vi "Go.vi"(9 "Timing Data":T1(array[cluster]), 10 "Control In":T2={"I-O.lvclass"=refnum, "Gantry"=refnum, "Dispenser"="COM1"}, 11 "Sensor Dispense in":refnum<class "Sensor Dispense.lvclass">) -> (2 "Control Out":T2={"I-O.lvclass"=refnum, "Gantry"=refnum, "Dispenser"="COM1"}, 3 "Sensor Dispense out":refnum<class "Sensor Dispense.lvclass">)   [LabVIEW 2021, in "Sensor Dispense.lvclass"]
uses:
  Sensor Dispense.lvclass
  C:/Users/HEP/Documents/GitHub/Gantry/UCSB-Gantry-HEP-main/Classes/Routine/Dispense/Dispense.lvclass
  Classes/Controller/Controllers.ctl
  Classes/Controller/I-O/I-O.lvclass
  C:/Program Files (x86)/Aerotech/A3200/LabVIEW/2010/Bin/Aerotech.A3200.dll
  Program Files (x86)/Aerotech/A3200/LabVIEW/2010/Bin/Aerotech.A3200.dll
  Sensor Dispense.lvclass/Sensor Dispense.ctl
  Classes/Controller/Motion/Motion.lvclass
  Classes/Controller/Dispenser/Dispenser.lvclass
  Classes/Controller/Motion/A3200/A3200.lvclass
  Classes/Controller/Controller.lvclass
panel:
  out "error out":errorcluster
  in  "error in (no error)":errorcluster
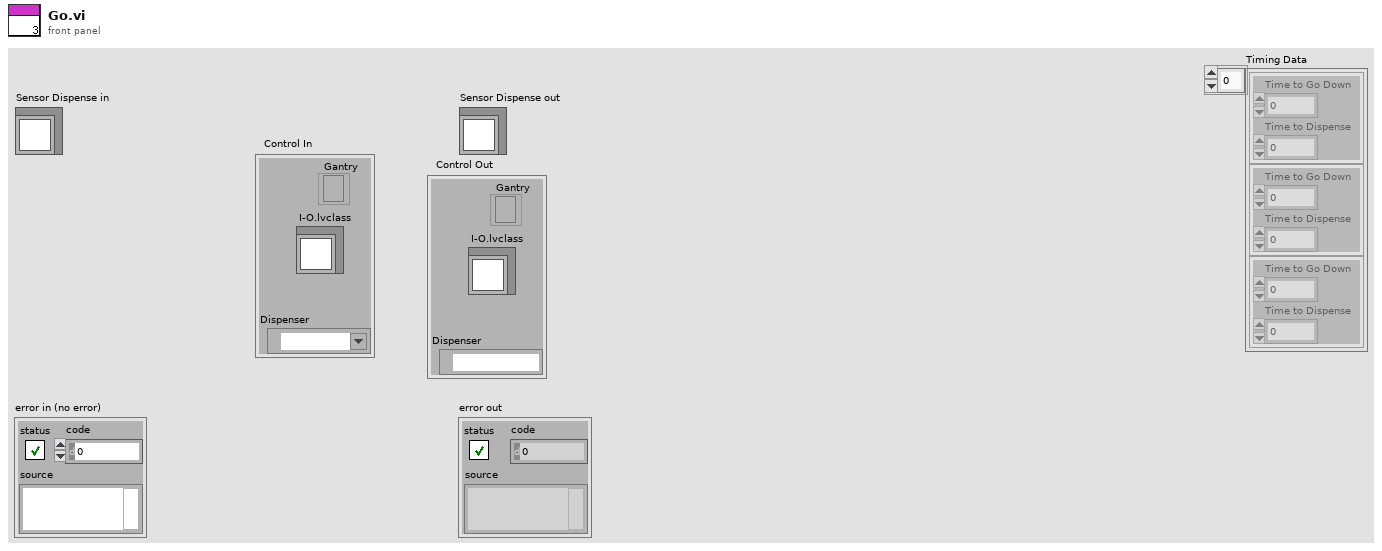
[diagram p1: front panel]
types:
  T1 = cluster{"Time to Go Down":i32, "Time to Dispense":i32}[]
  T2 = typedef "Controller.lvclass/Controllers.ctl" = cluster{"I-O.lvclass":refnum<class "I-O.lvclass">, "Gantry":refnum<k24>, "Dispenser":refnum<visa-resource-name>}
  T3 = cluster{"Endpoints":dbl[][], "Center":dbl[], "CW/CCW":dbl, "Dispense Type":enum16{"N-gon", "Square", "Arc", "Dot", "Line", "Circle"}}[]
  T4 = cluster{"Endpoints":dbl[][], "Center":dbl[], "CW/CCW":dbl, "Dispense Type":enum16{"N-gon", "Square", "Arc", "Dot", "Line", "Circle"}}
  T5 = enum16{"N-gon", "Square", "Arc", "Dot", "Line", "Circle"}
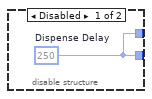
[diagram p2: hidden frame]
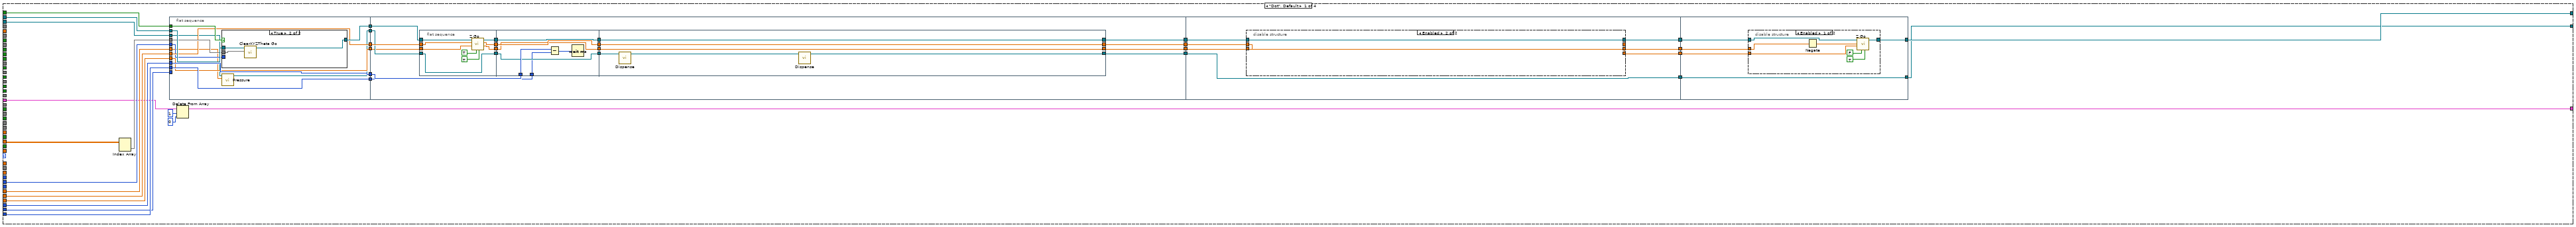
[diagram p4: hidden frame]
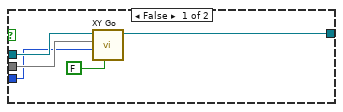
[diagram p5: hidden frame]
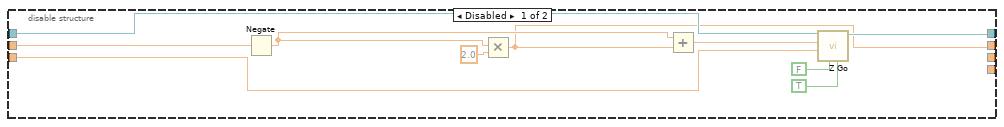
[diagram p6: hidden frame]
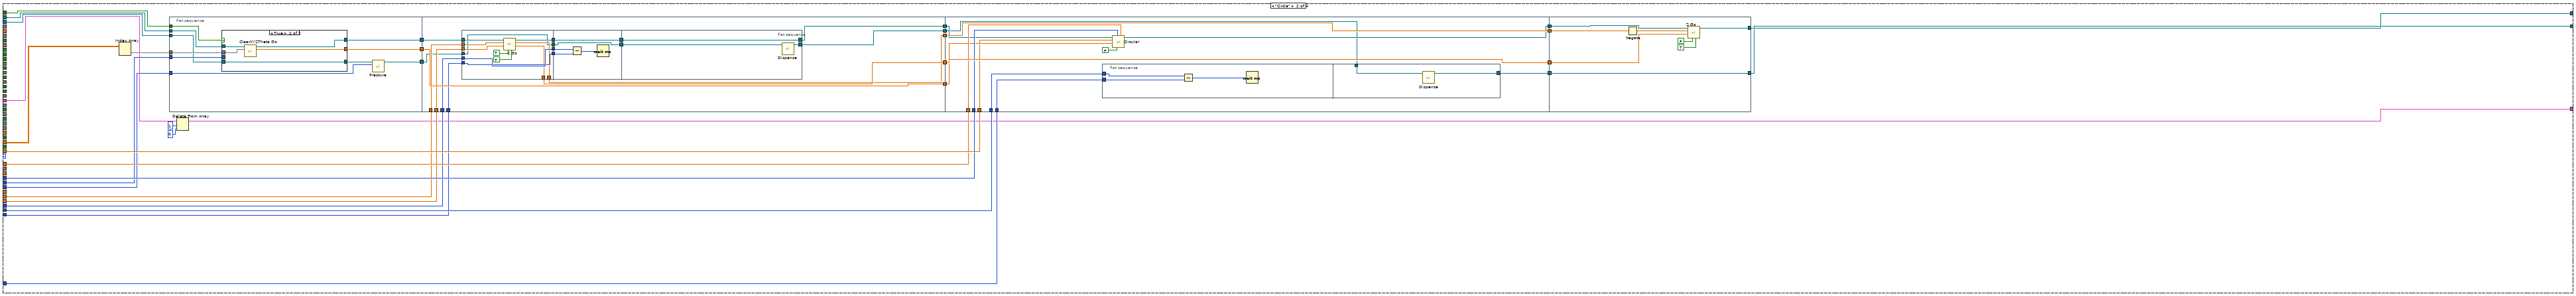
[diagram p8: hidden frame]
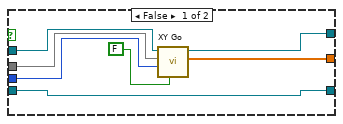
[diagram p9: hidden frame]
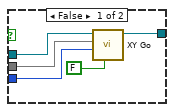
[diagram p10: hidden frame]
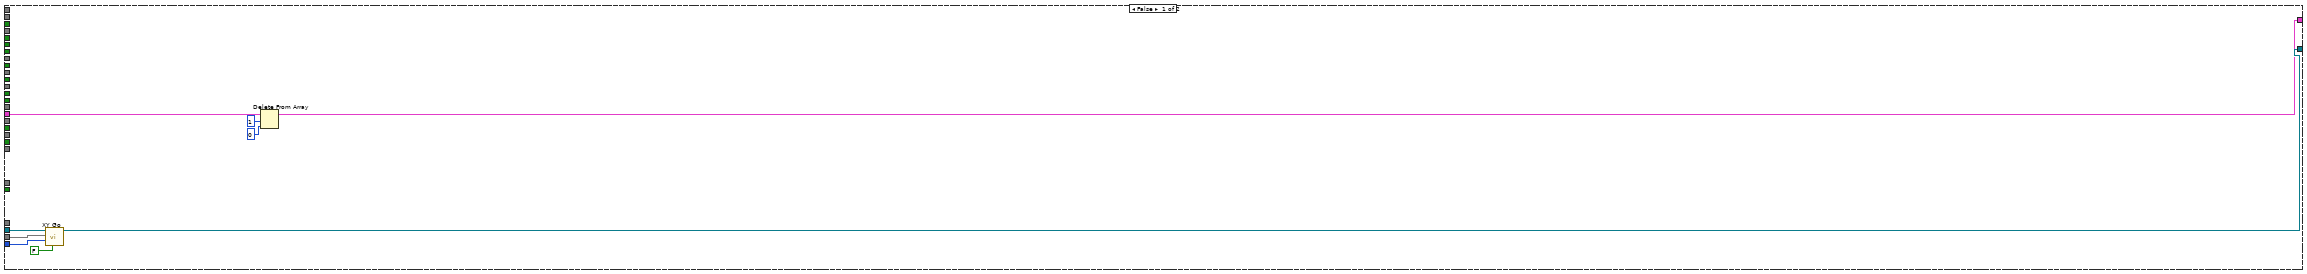
[diagram p11: hidden frame]
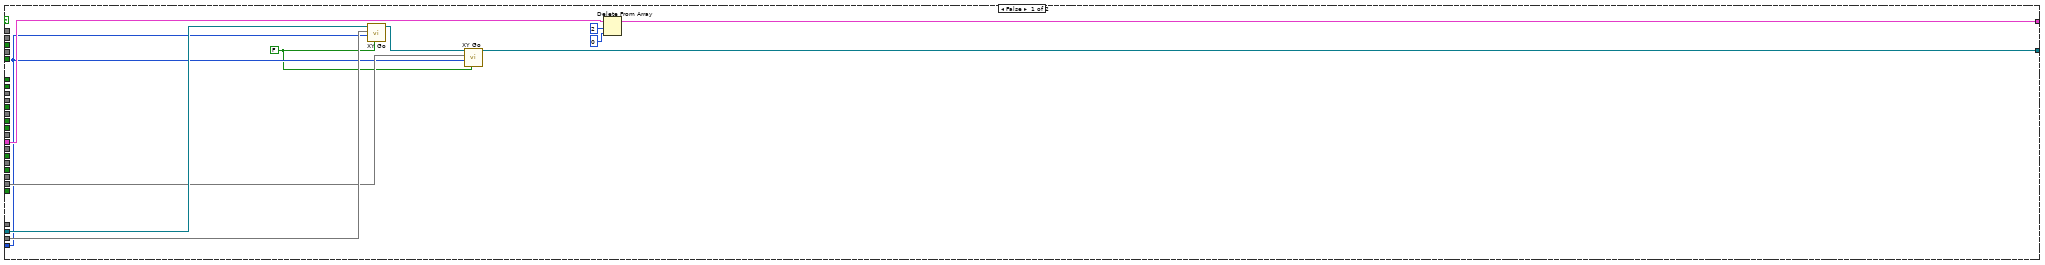
[diagram p12: hidden frame]
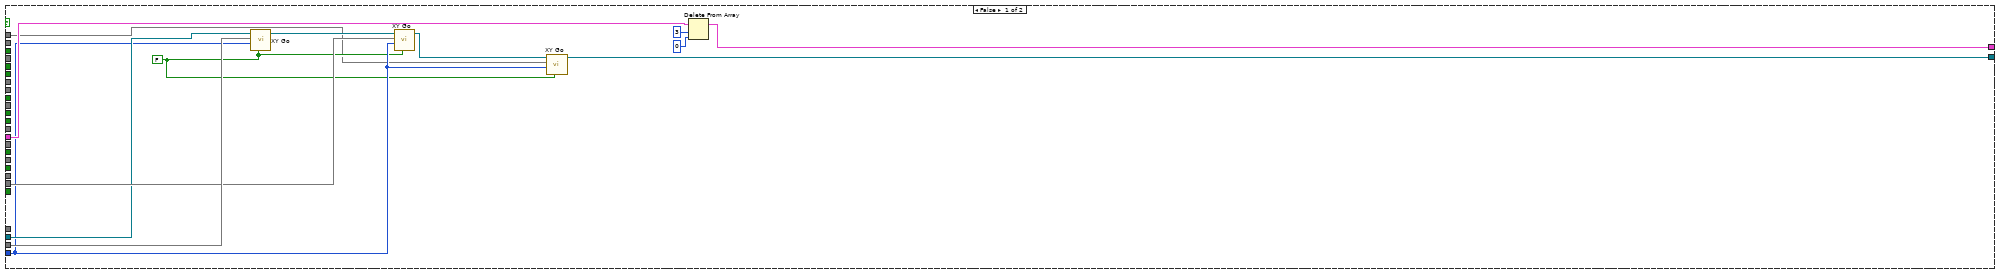
[diagram p13: hidden frame]
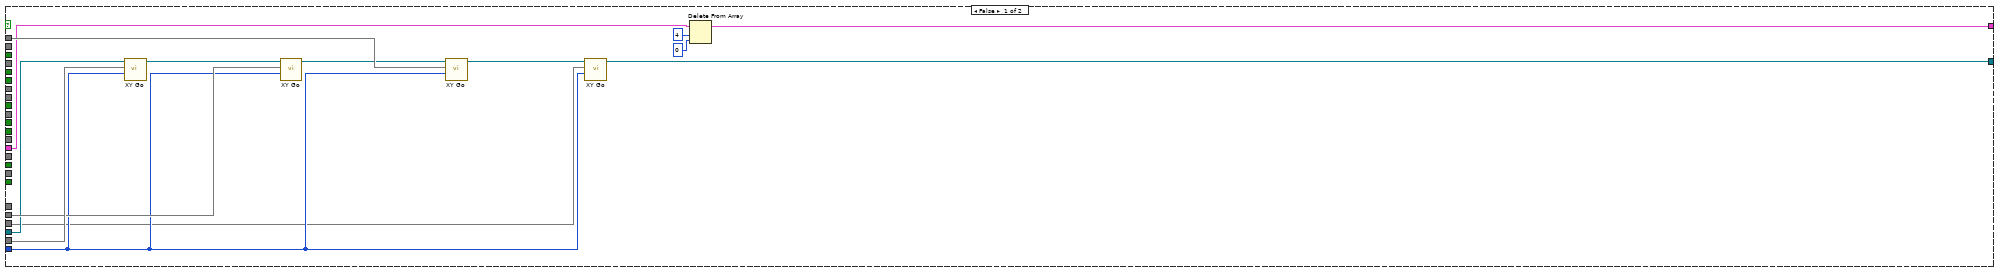
[diagram p14: hidden frame]
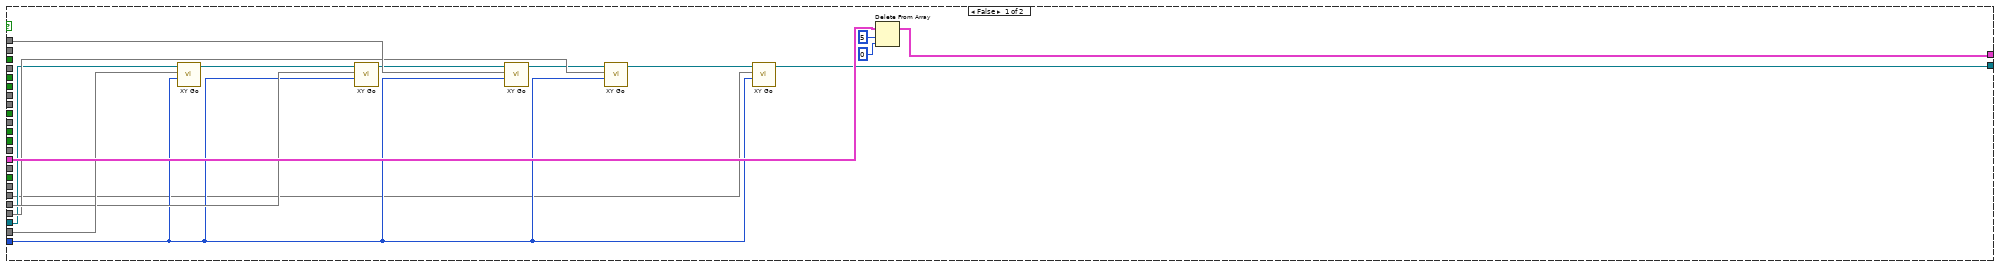
[diagram p15: hidden frame]
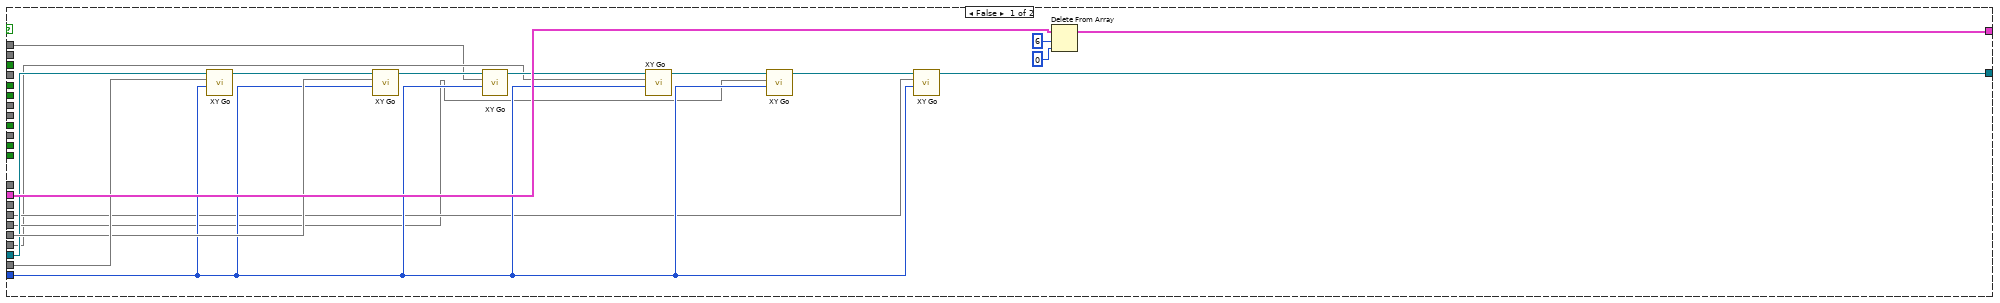
[diagram p16: hidden frame]
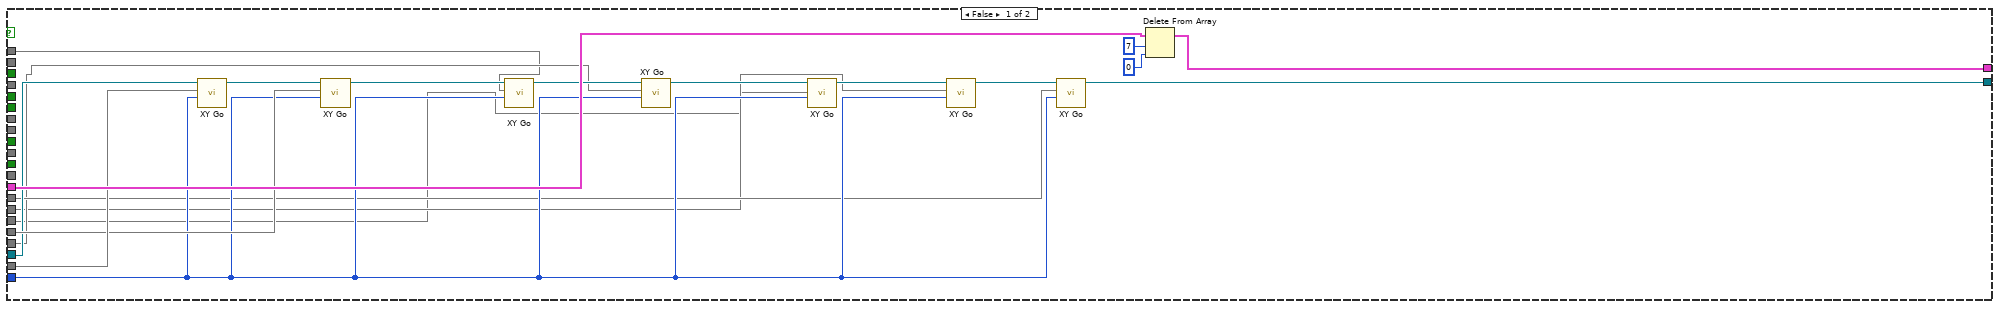
[diagram p17: hidden frame]
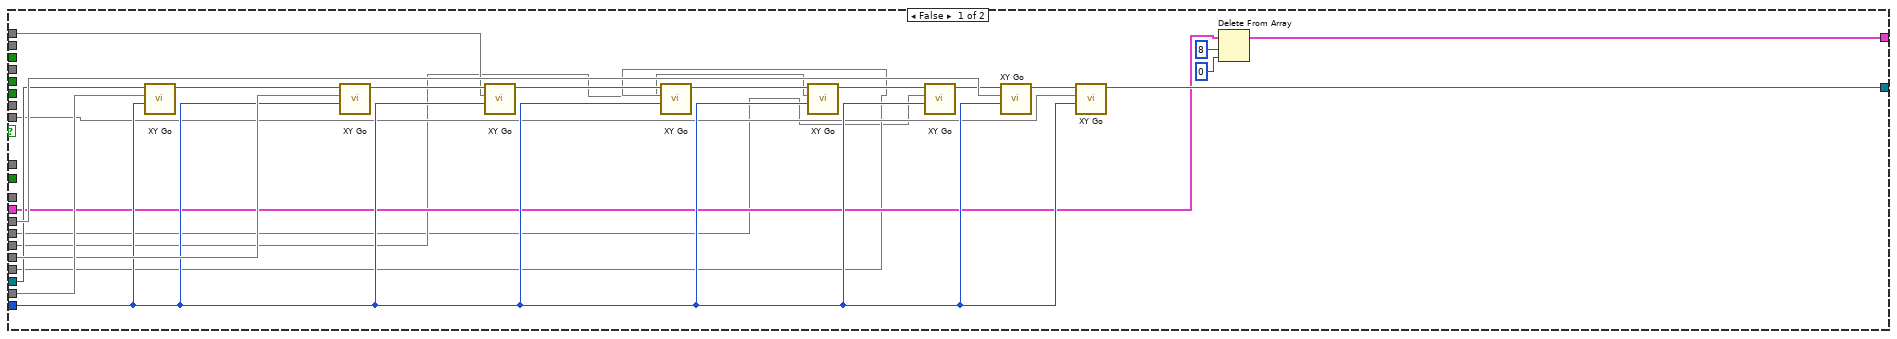
[diagram p18: hidden frame]
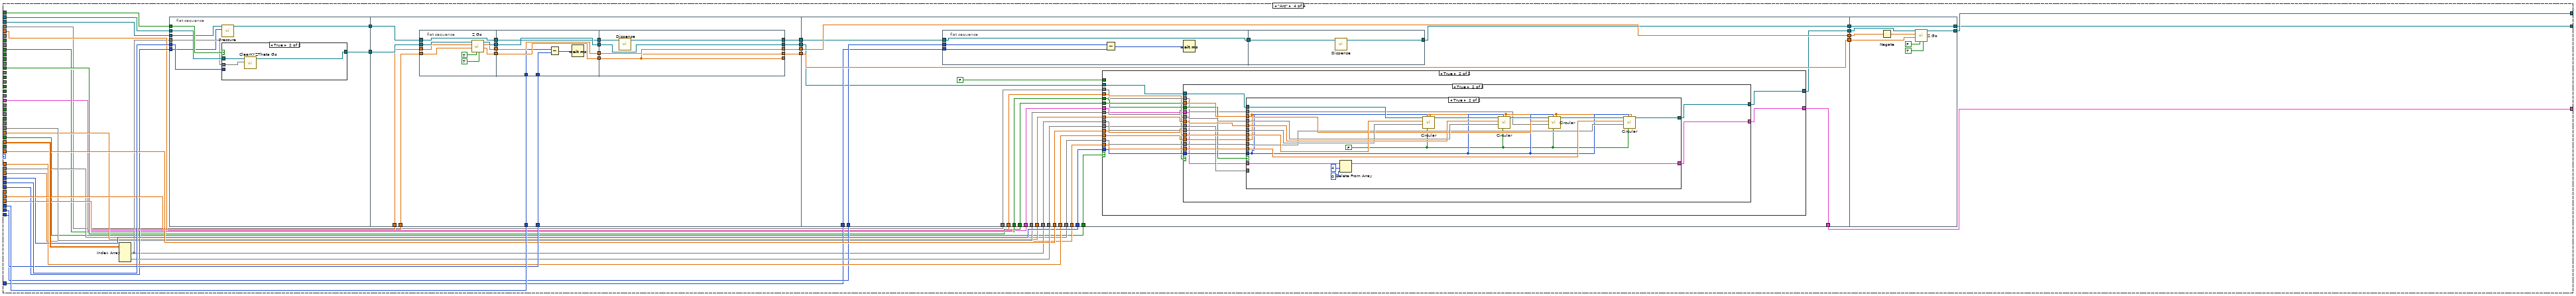
[diagram p19: hidden frame]
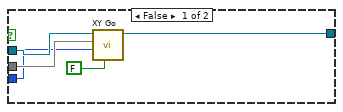
[diagram p20: hidden frame]
diagram:
  n1 = case shown="No Error" "error in (no error)" {
    selector: "error in (no error)" -> [w7 w1391]
    tunnel: "Sensor Dispense in" -> [w12 w1390]
    tunnel: [w11 w1390] -> w5
    tunnel: "Control In" -> [w10 w1389]
    tunnel: [w9 w1389] -> w3
    tunnel: [w8 w1391] -> w2
    frame No Error {
      n2 = in-place {
        in-place-border: w12 -> [w24]
        in-place-border: [w23] -> w11
        in-place-border: w7 -> [w17]
        in-place-border: [w16] -> w8
        n3 = in-place-cluster #1(w10) -> ("Gantry"=w25:refnum<k24>, "Dispenser"=w20:refnum<visa-resource-name>)
        n4 = Unbundle By Name(w24) -> ("Dispense Steps"=w21:T3, "Glue Speed"=w15:i32, "Move Speed"=w26:i32, "Line Pressure"=w13:i64, "Dot Pressure"=w14:dbl)
        n5 = while {
          tunnel: w26 -> [w167]
          shift-right: [w159] -> w22
          shift-left: w25 -> [w165]
          tunnel: w15 -> [w166]
          shift-right: [w151] -> w23
          shift-left: w24 -> [w163]
          shift-right: [w154] -> w18
          shift-left: w20 -> [w157]
          tunnel: "Timing Data" -> [w156] mode=indexing
          shift-right: [w147] -> w16
          shift-left: w17 -> [w147]
          tunnel: w14 -> [w149]
          tunnel: w13 -> [w148]
          shift-right: [w111] -> _
          shift-left: w21 -> [w63]
          i -> [w162]
          stop <- w113 stop-if-true
          # "740 is good"
          # "compares 3 and 4"
          # "compares 2 and 3"
          # "Compares 1 and 2"
          # "#2"
          # "#3"
          # "#4"
          # "#3"
          # "1/11/23 - Originally 750"
          n6 = Unbundle By Name(w156) -> ("Time to Go Down"=w155:i32, "Time to Dispense"=w145:i32)
          n7 = disable-structure shown="Enabled" {
            disable-tunnel: [w168 w172] -> w150
            disable-tunnel: [w168 w170] -> w146
            disable-tunnel: w145 -> [_ w171]
            frame Disabled {
              w168 = 250  # Dispense Delay
            }
            frame Enabled {
              w169 = 450  # End Dispense Delay
              w172 = 740  # Start Dispense Delay
              # "For arcs it is set to 250"
              # "525 - 1/23/2023"
              # "Originally 0"
              n8 = disable-structure shown="Disabled" {
                disable-tunnel: w171 -> [w177 _]
                disable-tunnel: [w174 w178] -> w170
                disable-tunnel: w169 -> [w173 w178]
                frame Disabled {
                  n9 = Less?(x=w177, y=w173) -> (x < y?=w176:bool)
                  n10 = Select(t=0, s=w176, f=w173) -> (s? t:f=w174:i32)
                }
                frame Enabled {
                }
              }
            }
          }
          n11 = Index Array(array=w63) -> (element=w143:T4)  [unwired: 1 in]
          n12 = Index Array(array=w63, index=11) -> (element=w69:T4)
          n13 = Index Array(array=w63, index=7) -> (element=w104:T4)
          n14 = Index Array(array=w63, index=9) -> (element=w75:T4)
          n15 = Index Array(array=w63, index=10) -> (element=w72:T4)
          n16 = Index Array(array=w63, index=12) -> (element=w66:T4)
          n17 = Index Array(array=w63, index=2) -> (element=w140:T4)
          n18 = Index Array(array=w63, index=8) -> (element=w78:T4)
          n19 = Index Array(array=w63, index=4) -> (element=w110:T4)
          n20 = Index Array(array=w63, index=6) -> (element=w106:T4)
          n21 = Index Array(array=w63, index=5) -> (element=w108:T4)
          n22 = Index Array(array=w63, index=1) -> (element=w142:T4)
          n23 = Index Array(array=w63, index=3) -> (element=w139:T4)
          n24 = Unbundle By Name(w140) -> ("Endpoints"=w137:dbl[][], "Center"=w118:dbl[])
          n25 = Unbundle By Name(w75) -> ("Endpoints"=w74:dbl[][])  [unwired: 1 out]
          n26 = Unbundle By Name(w104) -> ("Endpoints"=w103:dbl[][])  [unwired: 1 out]
          n27 = Unbundle By Name(w78) -> ("Endpoints"=w77:dbl[][])  [unwired: 1 out]
          n28 = Unbundle By Name(w110) -> ("Endpoints"=w109:dbl[][])  [unwired: 1 out]
          n29 = Unbundle By Name(w143) -> ("Endpoints"=w134:dbl[][], "Center"=w158:dbl[], "Dispense Type"=w160:T5, "CW/CCW"=w164:dbl)
          n30 = Unbundle By Name(w106) -> ("Endpoints"=w105:dbl[][])  [unwired: 1 out]
          n31 = Unbundle By Name(w139) -> ("Endpoints"=w138:dbl[][], "Center"=w117:dbl[])
          n32 = Unbundle By Name(w108) -> ("Endpoints"=w107:dbl[][])  [unwired: 1 out]
          n33 = Unbundle By Name(w142) -> ("Endpoints"=w141:dbl[][], "Center"=w119:dbl[])
          n34 = Unbundle By Name(w69) -> ("Endpoints"=w68:dbl[][])  [unwired: 1 out]
          n35 = Unbundle By Name(w72) -> ("Endpoints"=w71:dbl[][])  [unwired: 1 out]
          n36 = Unbundle By Name(w66) -> ("Endpoints"=w65:dbl[][])  [unwired: 1 out]
          n37 = Index Array(array=w103) -> (element #1=w82:dbl[], element #2=w61:dbl[])  [unwired: 4 in]
          n38 = Index Array(array=w137) -> (element #1=w131:dbl[], element #2=w27:dbl[])  [unwired: 4 in]
          n39 = Index Array(array=w107) -> (element #1=w93:dbl[], element #2=w31:dbl[])  [unwired: 4 in]
          n40 = Index Array(array=w138) -> (element #1=w130:dbl[], element #2=w28:dbl[])  [unwired: 4 in]
          n41 = Index Array(array=w77) -> (element #1=w62:dbl[], element #2=w55:dbl[])  [unwired: 4 in]
          n42 = Index Array(array=w74) -> (element #1=w56:dbl[], element #2=w49:dbl[])  [unwired: 4 in]
          n43 = Index Array(array=w109) -> (element #1=w98:dbl[], element #2=w30:dbl[])  [unwired: 4 in]
          n44 = Index Array(array=w105) -> (element #1=w88:dbl[], element #2=w29:dbl[])  [unwired: 4 in]
          n45 = Index Array(array=w141) -> (element #1=w132:dbl[], element #2=w120:dbl[])  [unwired: 4 in]
          n46 = Index Array(array=w68) -> (element #1=w43:dbl[], element #2=w38:dbl[])  [unwired: 4 in]
          n47 = Index Array(array=w71) -> (element #1=w50:dbl[], element #2=w44:dbl[])  [unwired: 4 in]
          n48 = Index Array(array=w65) -> (element #1=w37:dbl[], element #2=w32:dbl[])  [unwired: 4 in]
          n49 = Index Array(array=w134) -> (element #2=w133:dbl[])  [unwired: 4 in, 1 out]
          n50 = Equal?(x=w38, y=w37) -> (x = y?=w36:bool[])
          n51 = Equal?(x=w44, y=w43) -> (x = y?=w42:bool[])
          n52 = Equal?(x=w49, y=w50) -> (x = y?=w48:bool[])
          n53 = Equal?(x=w120, y=w131) -> (x = y?=w126:bool[])
          n54 = Equal?(x=w61, y=w62) -> (x = y?=w60:bool[])
          n55 = Equal?(x=w55, y=w56) -> (x = y?=w54:bool[])
          n56 = Equal?(x=w29, y=w82) -> (x = y?=w83:bool[])
          n57 = Equal?(x=w31, y=w88) -> (x = y?=w87:bool[])
          n58 = Equal?(x=w30, y=w93) -> (x = y?=w92:bool[])
          n59 = Equal?(x=w28, y=w98) -> (x = y?=w97:bool[])
          n60 = Equal?(x=w27, y=w130) -> (x = y?=w125:bool[])
          n61 = Index Array(array=w125) -> (element #1=w122:bool, element #2=w121:bool)  [unwired: 2 in]
          n62 = And(x=w122, y=w121) -> (x .and. y?=w114:bool)
          n63 = Index Array(array=w36) -> (element #1=w35:bool, element #2=w34:bool)  [unwired: 2 in]
          n64 = Equal?(x=w133, y=w132) -> (x = y?=w129:bool[])
          n65 = Index Array(array=w48) -> (element #1=w47:bool, element #2=w46:bool)  [unwired: 2 in]
          n66 = Index Array(array=w126) -> (element #1=w124:bool, element #2=w123:bool)  [unwired: 2 in]
          n67 = Index Array(array=w60) -> (element #1=w59:bool, element #2=w58:bool)  [unwired: 2 in]
          n68 = Index Array(array=w54) -> (element #1=w53:bool, element #2=w52:bool)  [unwired: 2 in]
          n69 = Index Array(array=w83) -> (element #1=w81:bool, element #2=w80:bool)  [unwired: 2 in]
          n70 = Index Array(array=w87) -> (element #1=w86:bool, element #2=w85:bool)  [unwired: 2 in]
          n71 = Index Array(array=w92) -> (element #1=w91:bool, element #2=w90:bool)  [unwired: 2 in]
          n72 = property on="Property Node" class="Sensor Dispense.lvclass"(reference=w163) -> (reference out=w151:refnum<class "Sensor Dispense.lvclass">, "Z height"=w153:dbl, "Z speed"=w152:dbl)  [unwired: 1 in, 1 out]
          n73 = Index Array(array=w42) -> (element #1=w41:bool, element #2=w40:bool)  [unwired: 2 in]
          n74 = Index Array(array=w97) -> (element #1=w96:bool, element #2=w95:bool)  [unwired: 2 in]
          n75 = And(x=w35, y=w34) -> (x .and. y?=w33:bool)
          n76 = Index Array(array=w129) -> (element #1=w128:bool, element #2=w127:bool)  [unwired: 2 in]
          n77 = And(x=w41, y=w40) -> (x .and. y?=w39:bool)
          n78 = And(x=w47, y=w46) -> (x .and. y?=w45:bool)
          n79 = And(x=w59, y=w58) -> (x .and. y?=w57:bool)
          n80 = And(x=w53, y=w52) -> (x .and. y?=w51:bool)
          n81 = And(x=w81, y=w80) -> (x .and. y?=w79:bool)
          n82 = And(x=w86, y=w85) -> (x .and. y?=w84:bool)
          n83 = And(x=w91, y=w90) -> (x .and. y?=w89:bool)
          n84 = And(x=w96, y=w95) -> (x .and. y?=w94:bool)
          n85 = And(x=w124, y=w123) -> (x .and. y?=w115:bool)
          n86 = And(x=w128, y=w127) -> (x .and. y?=w116:bool)
          n87 = Equal To 0?(x=w162) -> (x = 0?=w161:bool)
          n88 = case shown="\"Line\"" w160 {
            tunnel: w158 -> [_ w333 _ w1181]
            tunnel: w165 -> [w209 w334 w484 w1189]
            tunnel: w167 -> [w192 w327 w483 w1187]
            tunnel: [w208 w337 w480 w1177] -> w159
            tunnel: w166 -> [_ w332 w471 w1180]
            tunnel: w164 -> [_ w331 _ w1179]
            tunnel: w152 -> [w200 w329 w468 w1183]
            tunnel: w153 -> [w201 w330 w469 w1184]
            tunnel: w161 -> [w210 w328 w482 w1190]
            tunnel: w157 -> [w199 w311 w475 w1173]
            tunnel: w155 -> [w197 w318 w473 w1186]
            tunnel: w145 -> [w202 w319 w470 w1178]
            tunnel: w150 -> [w203 w317 w474 w1185]
            tunnel: [w207 w312 w478 w1176] -> w154
            tunnel: w134 -> [w206 w316 w477 w1188]
            tunnel: w149 -> [w191 _ _ _]
            tunnel: w148 -> [_ w309 w451 w1172]
            tunnel: w146 -> [_ w308 w450 w1171]
            tunnel: w120 -> [_ _ w447 w1170]
            tunnel: w119 -> [_ _ _ w1169]
            tunnel: w118 -> [_ _ _ w1168]
            tunnel: w117 -> [_ _ _ w1166]
            tunnel: w28 -> [_ _ w442 w1165]
            tunnel: w116 -> [_ _ w445 w1164]
            tunnel: w115 -> [_ _ w444 w1163]
            tunnel: w114 -> [_ _ w443 w1162]
            tunnel: w63 -> [w183 w307 w448 w1161]
            tunnel: [w180 w304 w449 w1160] -> w111
            tunnel: w27 -> [_ _ w446 w1159]
            tunnel: w94 -> [_ _ w441 _]
            tunnel: w30 -> [_ _ w440 _]
            tunnel: w89 -> [_ _ w439 _]
            tunnel: w31 -> [_ _ w438 _]
            tunnel: w84 -> [_ _ w437 _]
            tunnel: w79 -> [_ _ w436 _]
            tunnel: w29 -> [_ _ w435 _]
            tunnel: w61 -> [_ _ w434 _]
            tunnel: w57 -> [_ _ w433 _]
            tunnel: w55 -> [_ _ w432 _]
            tunnel: w51 -> [_ _ w431 _]
            tunnel: w49 -> [_ _ w430 _]
            tunnel: w45 -> [_ _ w429 _]
            tunnel: w44 -> [_ _ w428 _]
            tunnel: w39 -> [_ _ w427 _]
            tunnel: w38 -> [_ _ w426 _]
            tunnel: w33 -> [_ _ w425 _]
            tunnel: w32 -> [_ _ w424 _]
            frame "Dot", Default {
              n89 = Index Array(array=w206) -> (element=w205:dbl[])  [unwired: 2 in]
              n90 = flat-sequence {
                tunnel: w210 -> [w222]
                tunnel: w209 -> [w221]
                tunnel: w205 -> [w220]
                tunnel: [w219] -> w204
                tunnel: w203 -> [w216]
                tunnel: w202 -> [_]
                tunnel: w201 -> [w218]
                tunnel: w200 -> [w215]
                tunnel: w199 -> [w213]
                tunnel: [w218] -> w198
                tunnel: w197 -> [w217]
                tunnel: [w217] -> w196
                tunnel: [w216] -> w195
                tunnel: [w212] -> w194
                tunnel: [w215] -> w193
                tunnel: w192 -> [w214]
                tunnel: w191 -> [w211]
                tunnel: [w248] -> w188
                tunnel: w204 -> [w247]
                tunnel: [w244] -> w187
                tunnel: w198 -> [w243]
                tunnel: w196 -> [w242]
                tunnel: w195 -> [w241]
                tunnel: w194 -> [w240]
                tunnel: w193 -> [w237]
                tunnel: [w235] -> w186
                tunnel: [w234] -> w185
                tunnel: w188 -> [w276]
                tunnel: w187 -> [w275]
                tunnel: w186 -> [w274]
                tunnel: w185 -> [w273]
                tunnel: [w277] -> w190
                tunnel: [w276] -> w189
                tunnel: [w271] -> w184
                tunnel: [w272] -> w179
                tunnel: [w291] -> w207
                tunnel: [w294] -> w208
                tunnel: w190 -> [w295]
                tunnel: w189 -> [w291]
                tunnel: w184 -> [w293]
                tunnel: w179 -> [w292]
                frame #0 {
                  n91 = case shown="True" w222 {
                    tunnel: w221 -> [w227 w230]
                    tunnel: [w226 w229] -> w219
                    tunnel: w220 -> [w225 w228]
                    tunnel: w214 -> [w224 _]
                    frame False {
                      n92 = call "XY Go.vi"("return immediately"=FALSE, "Speed"=w224, "XY In"=w225, "Gantry In"=w227) -> ("Gantry Out"=w226:refnum<k24>)  [unwired: 5 in, 2 out]
                    }
                    frame True {
                      n93 = call "ClearXYZTheta Go.vi"("XYZTheta In"=w228, "Gantry In"=w230) -> ("Gantry Out"=w229:refnum<k24>)  [unwired: 7 in, 2 out]
                    }
                  }
                  n94 = call "Pressure.vi"("Pressure"=w211, "VISA resource name"=w213) -> ("VISA resource name out"=w212:refnum<visa-resource-name>)  [unwired: 8 in, 1 out]
                }
                frame #1 {
                  n95 = flat-sequence {
                    tunnel: w247 -> [w257]
                    tunnel: [w256] -> w245
                    tunnel: w243 -> [w250]
                    tunnel: w240 -> [w254]
                    tunnel: [w254] -> w239
                    tunnel: w237 -> [w253]
                    tunnel: [w252] -> w232
                    tunnel: [w249] -> w231
                    tunnel: [w264] -> w246
                    tunnel: w245 -> [w264]
                    tunnel: w242 -> [w263]
                    tunnel: w241 -> [w259]
                    tunnel: w239 -> [w262]
                    tunnel: [w262] -> w238
                    tunnel: [w261] -> w236
                    tunnel: [w260] -> w233
                    tunnel: w232 -> [w260]
                    tunnel: w231 -> [w261]
                    tunnel: [w270] -> w248
                    tunnel: w246 -> [w269]
                    tunnel: [w269] -> w244
                    tunnel: w238 -> [w268]
                    tunnel: w236 -> [w266]
                    tunnel: [w266] -> w235
                    tunnel: [w265] -> w234
                    tunnel: w233 -> [w265]
                    frame #0 {
                      n96 = call "Z Go.vi"("Increment"=TRUE, "Return Immediately"=TRUE, "Speed In"=w253, "Position In"=w250, "Gantry In"=w257) -> ("Speed Out"=w252:dbl, "Position Out"=w249:dbl, "Gantry Out"=w256:refnum<k24>)  [unwired: 3 in, 1 out]
                    }
                    frame #1 {
                      n97 = Subtract(x=w263, y=w259) -> (x-y=w258:i32)
                      n98 = Wait (ms)(milliseconds to wait=w258) -> ()  [unwired: 1 out]
                    }
                    frame #2 {
                      n99 = call "Dispense.vi"("Dispenser In"=w268) -> ("Dispenser Out"=w267:refnum<visa-resource-name>)  [unwired: 9 in, 1 out]
                      n100 = call "Dispense.vi"("Dispenser In"=w267) -> ("Dispenser Out"=w270:refnum<visa-resource-name>)  [unwired: 9 in, 1 out]
                    }
                  }
                }
                frame #2 {
                  n101 = disable-structure shown="Enabled" {
                    disable-tunnel: [w287 w290] -> w277
                    disable-tunnel: w275 -> [w286 w290]
                    disable-tunnel: w274 -> [w285 w288]
                    disable-tunnel: w273 -> [w282 w289]
                    disable-tunnel: [w278 _] -> _
                    disable-tunnel: [_ w289] -> w272
                    disable-tunnel: [_ w288] -> w271
                    frame Disabled {
                      n102 = Negate(x=w285) -> (-x=w280:dbl)
                      n103 = Multiply(x=w280, y=2.0) -> (x*y=w278:dbl)
                      n104 = Add(x=w280, y=w278) -> (x+y=w281:dbl)
                      n105 = call "Z Go.vi"("Increment"=TRUE, "Return Immediately"=FALSE, "Speed In"=w282, "Position In"=w281, "Gantry In"=w286) -> ("Gantry Out"=w287:refnum<k24>)  [unwired: 3 in, 3 out]
                    }
                    frame Enabled {
                    }
                  }
                }
                frame #3 {
                  n106 = disable-structure shown="Enabled" {
                    disable-tunnel: w295 -> [w302 w303]
                    disable-tunnel: [w301 w303] -> w294
                    disable-tunnel: w293 -> [w296 _]
                    disable-tunnel: w292 -> [w297 _]
                    frame Enabled {
                      n107 = Negate(x=w296) -> (-x=w300:dbl)
                      n108 = call "Z Go.vi"("Increment"=TRUE, "Return Immediately"=FALSE, "Speed In"=w297, "Position In"=w300, "Gantry In"=w302) -> ("Gantry Out"=w301:refnum<k24>)  [unwired: 3 in, 3 out]
                    }
                    frame Disabled {
                    }
                  }
                }
              }
              n109 = Delete From Array(array=w183, length=1, index=0) -> (array with subset deleted=w180:T3)  [unwired: 1 out]
            }
            frame "Circle" {
              n110 = Index Array(array=w316) -> (element=w315:dbl[])  [unwired: 2 in]
              n111 = flat-sequence {
                tunnel: [w345] -> w336
                tunnel: w334 -> [w346]
                tunnel: w328 -> [w347]
                tunnel: w327 -> [w344]
                tunnel: [w343] -> w325
                tunnel: w315 -> [w342]
                tunnel: w311 -> [w341]
                tunnel: [w339] -> w310
                tunnel: w309 -> [w338]
                tunnel: w330 -> [w369]
                tunnel: w329 -> [w370]
                tunnel: [w376] -> w326
                tunnel: [w367] -> w324
                tunnel: [w368] -> w323
                tunnel: w325 -> [w376]
                tunnel: w336 -> [w366]
                tunnel: [w375] -> w320
                tunnel: w318 -> [w374]
                tunnel: w317 -> [w373]
                tunnel: [w363] -> w314
                tunnel: w310 -> [w362]
                tunnel: [w398] -> w335
                tunnel: [w408] -> w322
                tunnel: [w407] -> w321
                tunnel: w319 -> [w406]
                tunnel: w320 -> [w396]
                tunnel: w326 -> [w401]
                tunnel: w324 -> [w408]
                tunnel: w323 -> [w407]
                tunnel: w331 -> [w404]
                tunnel: w332 -> [w402]
                tunnel: w333 -> [w400]
                tunnel: w314 -> [w399]
                tunnel: [w405] -> w313
                tunnel: w308 -> [w397]
                tunnel: [w419] -> w337
                tunnel: w335 -> [w420]
                tunnel: w322 -> [w421]
                tunnel: w321 -> [w418]
                tunnel: w313 -> [w417]
                tunnel: [w417] -> w312
                frame #0 {
                  n112 = case shown="True" w347 {
                    tunnel: w346 -> [w354 w359]
                    tunnel: [w353 w358] -> w345
                    tunnel: w344 -> [w352 _]
                    tunnel: [w351 w356] -> w343
                    tunnel: w342 -> [w350 w357]
                    tunnel: w341 -> [w349 w355]
                    tunnel: [w349 w355] -> w340
                    frame False {
                      n113 = call "XY Go.vi"("return immediately"=FALSE, "Speed"=w352, "XY In"=w350, "Gantry In"=w354) -> ("XY Out"=w351:dbl[], "Gantry Out"=w353:refnum<k24>)  [unwired: 5 in, 1 out]
                    }
                    frame True {
                      n114 = call "ClearXYZTheta Go.vi"("XYZTheta In"=w357, "Gantry In"=w359) -> ("XYZTheta Out"=w356:dbl[], "Gantry Out"=w358:refnum<k24>)  [unwired: 7 in, 1 out]
                    }
                  }
                  n115 = call "Pressure.vi"("Pressure"=w338, "VISA resource name"=w340) -> ("VISA resource name out"=w339:refnum<visa-resource-name>)  [unwired: 8 in, 1 out]
                }
                frame #1 {
                  n116 = flat-sequence {
                    tunnel: w373 -> [w386]
                    tunnel: w374 -> [w387]
                    tunnel: [w387] -> w372
                    tunnel: [w386] -> w371
                    tunnel: w370 -> [w385]
                    tunnel: w369 -> [w384]
                    tunnel: [w383] -> w368
                    tunnel: [w382] -> w367
                    tunnel: w366 -> [w381]
                    tunnel: [w380] -> w365
                    tunnel: w362 -> [w378]
                    tunnel: [w378] -> w361
                    tunnel: w372 -> [w392]
                    tunnel: w371 -> [w391]
                    tunnel: w365 -> [w390]
                    tunnel: [w390] -> w364
                    tunnel: w361 -> [w389]
                    tunnel: [w389] -> w360
                    tunnel: [w395] -> w375
                    tunnel: w364 -> [w394]
                    tunnel: [w394] -> w363
                    tunnel: w360 -> [w393]
                    frame #0 {
                      n117 = call "Z Go.vi"("Increment"=TRUE, "Return Immediately"=TRUE ("return immediately"), "Speed In"=w385, "Position In"=w384, "Gantry In"=w381) -> ("Speed Out"=w383:dbl, "Position Out"=w382:dbl, "Gantry Out"=w380:refnum<k24>)  [unwired: 3 in, 1 out]
                    }
                    frame #1 {
                      n118 = Subtract(x=w392, y=w391) -> (x-y=w388:i32)
                      n119 = Wait (ms)(milliseconds to wait=w388) -> ()  [unwired: 1 out]
                    }
                    frame #2 {
                      n120 = call "Dispense.vi"("Dispenser In"=w393) -> ("Dispenser Out"=w395:refnum<visa-resource-name>)  [unwired: 9 in, 1 out]
                    }
                  }
                }
                frame #2 {
                  n121 = flat-sequence {
                    tunnel: w406 -> [w411]
                    tunnel: w397 -> [w409]
                    tunnel: [w413] -> w405
                    tunnel: w396 -> [w412]
                    frame #0 {
                      n122 = Subtract(x=w411, y=w409) -> (x-y=w410:i32)
                      n123 = Wait (ms)(milliseconds to wait=w410) -> ()  [unwired: 1 out]
                    }
                    frame #1 {
                      n124 = call "Dispense.vi"("Dispenser In"=w412) -> ("Dispenser Out"=w413:refnum<visa-resource-name>)  [unwired: 9 in, 1 out]
                    }
                  }
                  n125 = call "Circular.vi"("Direction"=w404, "return immediately"=FALSE, "Speed"=w402, "XY End"=w401, "XY Center"=w400, "Gantry In"=w399) -> ("Gantry Out"=w398:refnum<k24>)  [unwired: 4 in, 1 out]
                }
                frame #3 {
                  n126 = Negate(x=w421) -> (-x=w416:dbl)
                  n127 = call "Z Go.vi"("Increment"=TRUE, "Return Immediately"=FALSE, "Speed In"=w418, "Position In"=w416, "Gantry In"=w420) -> ("Gantry Out"=w419:refnum<k24>)  [unwired: 3 in, 3 out]
                }
              }
              n128 = Delete From Array(array=w307, length=1, index=0) -> (array with subset deleted=w304:T3)  [unwired: 1 out]
            }
            frame "Line" {
              n129 = Index Array(array=w477) -> (element #1=w476:dbl[], element #2=w472:dbl[])  [unwired: 4 in]
              n130 = flat-sequence {
                tunnel: w484 -> [w499]
                tunnel: w483 -> [w498]
                tunnel: w482 -> [w497]
                tunnel: [w496] -> w481
                tunnel: w476 -> [w495]
                tunnel: w475 -> [w487]
                tunnel: w474 -> [w491]
                tunnel: w473 -> [w492]
                tunnel: w472 -> [w490]
                tunnel: w471 -> [w489]
                tunnel: w470 -> [w488]
                tunnel: w469 -> [w494]
                tunnel: w468 -> [w493]
                tunnel: [w494] -> w467
                tunnel: [w493] -> w466
                tunnel: [w492] -> w464
                tunnel: [w491] -> w463
                tunnel: [w486] -> w462
                tunnel: [w490] -> w460
                tunnel: [w489] -> w458
                tunnel: [w488] -> w456
                tunnel: w451 -> [w485]
                tunnel: w481 -> [w531]
                tunnel: w467 -> [w530]
                tunnel: w466 -> [w529]
                tunnel: [w526] -> w465
                tunnel: w464 -> [w523]
                tunnel: w463 -> [w524]
                tunnel: w462 -> [w525]
                tunnel: [w537] -> w461
                tunnel: w460 -> [w536]
                tunnel: [w535] -> w459
                tunnel: w458 -> [w534]
                tunnel: [w532] -> w457
                tunnel: w456 -> [w533]
                tunnel: [w528] -> w453
                tunnel: [w527] -> w423
                tunnel: [w508] -> w422
                tunnel: [w611] -> w479
                tunnel: w465 -> [w600]
                tunnel: w461 -> [w601]
                tunnel: w459 -> [w602]
                tunnel: w457 -> [w609]
                tunnel: [w599] -> w455
                tunnel: [w608] -> w454
                tunnel: w453 -> [w606]
                tunnel: [w605] -> w452
                tunnel: w450 -> [w598]
                tunnel: [w597] -> w449
                tunnel: w448 -> [w596]
                tunnel: w447 -> [w595]
                tunnel: w446 -> [w594]
                tunnel: w445 -> [w593]
                tunnel: w444 -> [w592]
                tunnel: w443 -> [w591]
                tunnel: w442 -> [w590]
                tunnel: w441 -> [w589]
                tunnel: w440 -> [w588]
                tunnel: w439 -> [w587]
                tunnel: w438 -> [w586]
                tunnel: w437 -> [w585]
                tunnel: w436 -> [w584]
                tunnel: w435 -> [w583]
                tunnel: w434 -> [w582]
                tunnel: w433 -> [w581]
                tunnel: w432 -> [w580]
                tunnel: w431 -> [w579]
                tunnel: w430 -> [w578]
                tunnel: w429 -> [w577]
                tunnel: w428 -> [w576]
                tunnel: w427 -> [w575]
                tunnel: w426 -> [w574]
                tunnel: w425 -> [w573]
                tunnel: w424 -> [w572]
                tunnel: w423 -> [w603]
                tunnel: w422 -> [w571]
                tunnel: [w1158] -> w480
                tunnel: w479 -> [w1157]
                tunnel: [w1157] -> w478
                tunnel: w455 -> [w1156]
                tunnel: w454 -> [w1155]
                tunnel: w452 -> [w1153]
                frame #0 {
                  n131 = case shown="True" w497 {
                    tunnel: w499 -> [w504 w507]
                    tunnel: w498 -> [w503 _]
                    tunnel: [w502 w506] -> w496
                    tunnel: w495 -> [w501 w505]
                    frame False {
                      n132 = call "XY Go.vi"("return immediately"=FALSE, "Speed"=w503, "XY In"=w501, "Gantry In"=w504) -> ("Gantry Out"=w502:refnum<k24>)  [unwired: 5 in, 2 out]
                    }
                    frame True {
                      n133 = call "ClearXYZTheta Go.vi"("XYZTheta In"=w505, "Gantry In"=w507) -> ("Gantry Out"=w506:refnum<k24>)  [unwired: 7 in, 2 out]
                    }
                  }
                  n134 = call "Pressure.vi"("Pressure"=w485, "VISA resource name"=w487) -> ("VISA resource name out"=w486:refnum<visa-resource-name>)  [unwired: 8 in, 1 out]
                }
                frame #1 {
                  n135 = flat-sequence {
                    tunnel: w523 -> [w546]
                    tunnel: w524 -> [w538]
                    tunnel: w536 -> [w545]
                    tunnel: w534 -> [w544]
                    tunnel: w533 -> [w543]
                    tunnel: w531 -> [w554]
                    tunnel: w530 -> [w553]
                    tunnel: w529 -> [w552]
                    tunnel: w525 -> [w540]
                    tunnel: [w546] -> w522
                    tunnel: [w538] -> w521
                    tunnel: [w545] -> w520
                    tunnel: [w544] -> w519
                    tunnel: [w543] -> w518
                    tunnel: [w549] -> w517
                    tunnel: [w548] -> w516
                    tunnel: [w547] -> w515
                    tunnel: [w541] -> w508
                    tunnel: w522 -> [_]
                    tunnel: w521 -> [_]
                    tunnel: w520 -> [w564]
                    tunnel: w519 -> [w563]
                    tunnel: w518 -> [w562]
                    tunnel: w517 -> [w561]
                    tunnel: w516 -> [w560]
                    tunnel: w515 -> [w559]
                    tunnel: [w564] -> w514
                    tunnel: [w563] -> w513
                    tunnel: [w562] -> w512
                    tunnel: [w561] -> w511
                    tunnel: [w560] -> w510
                    tunnel: [w559] -> w509
                    tunnel: [w570] -> w537
                    tunnel: [w569] -> w535
                    tunnel: [w568] -> w532
                    tunnel: [w567] -> w528
                    tunnel: [w566] -> w527
                    tunnel: [w565] -> w526
                    tunnel: w514 -> [w570]
                    tunnel: w513 -> [w569]
                    tunnel: w512 -> [w568]
                    tunnel: w511 -> [w567]
                    tunnel: w510 -> [w566]
                    tunnel: w509 -> [w565]
                    frame #0 {
                      n136 = call "Z Go.vi"("Increment"=TRUE ("Return Immediately"), "Return Immediately"=FALSE ("Increment"), "Speed In"=w552, "Position In"=w553, "Gantry In"=w554) -> ("Speed Out"=w548:dbl, "Position Out"=w549:dbl, "Gantry Out"=w547:refnum<k24>)  [unwired: 3 in, 1 out]
                      n137 = Subtract(x=w546, y=w538) -> (x-y=w542:i32)
                      n138 = flat-sequence {
                        tunnel: w542 -> [w556]
                        tunnel: w540 -> [w555]
                        tunnel: [w555] -> w539
                        tunnel: [w558] -> w541
                        tunnel: w539 -> [w557]
                        frame #0 {
                          n139 = Wait (ms)(milliseconds to wait=w556) -> ()  [unwired: 1 out]
                        }
                        frame #1 {
                          n140 = call "Dispense.vi"("Dispenser In"=w557) -> ("Dispenser Out"=w558:refnum<visa-resource-name>)  [unwired: 9 in, 1 out]
                        }
                      }
                    }
                    frame #1 {
                    }
                    frame #2 {
                    }
                  }
                }
                frame #2 {
                  n141 = case shown="True" w593 {
                    tunnel: w602 -> [w620 w645]
                    tunnel: w601 -> [w619 w648]
                    tunnel: w600 -> [w618 w647]
                    tunnel: [w617 w644] -> w599
                    tunnel: [w614 w643] -> w597
                    tunnel: w596 -> [w615 w649]
                    tunnel: w595 -> [_ w646]
                    tunnel: w594 -> [_ w642]
                    tunnel: w592 -> [_ w641]
                    tunnel: w591 -> [_ w640]
                    tunnel: w590 -> [_ w639]
                    tunnel: w589 -> [_ w638]
                    tunnel: w588 -> [_ w637]
                    tunnel: w587 -> [_ w636]
                    tunnel: w586 -> [_ w635]
                    tunnel: w585 -> [_ w634]
                    tunnel: w584 -> [_ w633]
                    tunnel: w583 -> [_ w632]
                    tunnel: w582 -> [_ w631]
                    tunnel: w581 -> [_ w630]
                    tunnel: w580 -> [_ w629]
                    tunnel: w579 -> [_ w628]
                    tunnel: w578 -> [_ w627]
                    tunnel: w577 -> [_ w626]
                    tunnel: w576 -> [_ w625]
                    tunnel: w575 -> [_ w624]
                    tunnel: w574 -> [_ w623]
                    tunnel: w573 -> [_ w622]
                    tunnel: w572 -> [_ w621]
                    frame False {
                      n142 = call "XY Go.vi"("return immediately"=FALSE, "Speed"=w620, "XY In"=w619, "Gantry In"=w618) -> ("Gantry Out"=w617:refnum<k24>)  [unwired: 5 in, 2 out]
                      n143 = Delete From Array(array=w615, length=1, index=0) -> (array with subset deleted=w614:T3)  [unwired: 1 out]
                    }
                    frame True {
                      # "#7"
                      # "#2"
                      # "#1"
                      n144 = case shown="True" w641 {
                        tunnel: w649 -> [w660 w688]
                        tunnel: w648 -> [w657 w686]
                        tunnel: w647 -> [w656 w684]
                        tunnel: w646 -> [w654 w685]
                        tunnel: w645 -> [w653 w682]
                        tunnel: [w652 w683] -> w644
                        tunnel: [w651 w687] -> w643
                        tunnel: w642 -> [_ w681]
                        tunnel: w640 -> [_ w680]
                        tunnel: w639 -> [_ w679]
                        tunnel: w638 -> [_ w678]
                        tunnel: w637 -> [_ w677]
                        tunnel: w636 -> [_ w676]
                        tunnel: w635 -> [_ w675]
                        tunnel: w634 -> [_ w674]
                        tunnel: w633 -> [_ w673]
                        tunnel: w632 -> [_ w672]
                        tunnel: w631 -> [_ w671]
                        tunnel: w630 -> [_ w670]
                        tunnel: w629 -> [_ w669]
                        tunnel: w628 -> [_ w668]
                        tunnel: w627 -> [_ w667]
                        tunnel: w626 -> [_ w666]
                        tunnel: w625 -> [_ w665]
                        tunnel: w624 -> [_ w664]
                        tunnel: w623 -> [_ w663]
                        tunnel: w622 -> [_ w662]
                        tunnel: w621 -> [_ w661]
                        frame False {
                          w650 = FALSE ("return immediately")
                          n145 = call "XY Go.vi"("return immediately"=w650, "Speed"=w653, "XY In"=w657, "Gantry In"=w656) -> ("Gantry Out"=w655:refnum<k24>)  [unwired: 5 in, 2 out]
                          n146 = call "XY Go.vi"("return immediately"=w650, "Speed"=w653, "XY In"=w654, "Gantry In"=w655) -> ("Gantry Out"=w652:refnum<k24>)  [unwired: 5 in, 2 out]
                          n147 = Delete From Array(array=w660, length=2, index=0) -> (array with subset deleted=w651:T3)  [unwired: 1 out]
                        }
                        frame True {
                          # "#9"
                          # "#8"
                          # "#3"
                          # "#4"
                          # "#7"
                          n148 = case shown="True" w680 {
                            tunnel: w688 -> [w701 w722]
                            tunnel: [w698 w721] -> w687
                            tunnel: w686 -> [w697 w728]
                            tunnel: w685 -> [w696 w727]
                            tunnel: w684 -> [w695 w724]
                            tunnel: [w692 w723] -> w683
                            tunnel: w682 -> [w691 w725]
                            tunnel: w681 -> [w689 w726]
                            tunnel: w679 -> [_ w720]
                            tunnel: w678 -> [_ w719]
                            tunnel: w677 -> [_ w718]
                            tunnel: w676 -> [_ w717]
                            tunnel: w675 -> [_ w716]
                            tunnel: w674 -> [_ w715]
                            tunnel: w673 -> [_ w714]
                            tunnel: w672 -> [_ w713]
                            tunnel: w671 -> [_ w712]
                            tunnel: w670 -> [_ w711]
                            tunnel: w669 -> [_ w710]
                            tunnel: w668 -> [_ w709]
                            tunnel: w667 -> [_ w708]
                            tunnel: w666 -> [_ w707]
                            tunnel: w665 -> [_ w706]
                            tunnel: w664 -> [_ w705]
                            tunnel: w663 -> [_ w704]
                            tunnel: w662 -> [_ w703]
                            tunnel: w661 -> [_ w702]
                            frame False {
                              w690 = FALSE ("return immediately")
                              n149 = call "XY Go.vi"("return immediately"=w690, "Speed"=w691, "XY In"=w697, "Gantry In"=w695) -> ("Gantry Out"=w694:refnum<k24>)  [unwired: 5 in, 2 out]
                              n150 = call "XY Go.vi"("return immediately"=w690, "Speed"=w691, "XY In"=w696, "Gantry In"=w694) -> ("Gantry Out"=w693:refnum<k24>)  [unwired: 5 in, 2 out]
                              n151 = call "XY Go.vi"("return immediately"=w690, "Speed"=w691, "XY In"=w689, "Gantry In"=w693) -> ("Gantry Out"=w692:refnum<k24>)  [unwired: 5 in, 2 out]
                              n152 = Delete From Array(array=w701, length=3, index=0) -> (array with subset deleted=w698:T3)  [unwired: 1 out]
                            }
                            frame True {
                              # "#5"
                              # "#6"
                              n153 = case shown="True" w719 {
                                tunnel: w728 -> [w742 w766]
                                tunnel: w727 -> [w741 w765]
                                tunnel: w726 -> [w740 w764]
                                tunnel: w725 -> [w739 w762]
                                tunnel: w724 -> [w738 w761]
                                tunnel: [w734 w760] -> w723
                                tunnel: w722 -> [w731 w768]
                                tunnel: [w730 w767] -> w721
                                tunnel: w720 -> [w729 w763]
                                tunnel: w718 -> [_ w759]
                                tunnel: w717 -> [_ w758]
                                tunnel: w716 -> [_ w743]
                                tunnel: w715 -> [_ w757]
                                tunnel: w714 -> [_ w756]
                                tunnel: w713 -> [_ w755]
                                tunnel: w712 -> [_ w754]
                                tunnel: w711 -> [_ w753]
                                tunnel: w710 -> [_ w752]
                                tunnel: w709 -> [_ w751]
                                tunnel: w708 -> [_ w750]
                                tunnel: w707 -> [_ w749]
                                tunnel: w706 -> [_ w748]
                                tunnel: w705 -> [_ w747]
                                tunnel: w704 -> [_ w746]
                                tunnel: w703 -> [_ w745]
                                tunnel: w702 -> [_ w744]
                                frame False {
                                n154 = call "XY Go.vi"("Speed"=w739, "XY In"=w742, "Gantry In"=w738) -> ("Gantry Out"=w737:refnum<k24>)  [unwired: 6 in, 2 out]
                                n155 = call "XY Go.vi"("Speed"=w739, "XY In"=w741, "Gantry In"=w737) -> ("Gantry Out"=w736:refnum<k24>)  [unwired: 6 in, 2 out]
                                n156 = call "XY Go.vi"("Speed"=w739, "XY In"=w740, "Gantry In"=w736) -> ("Gantry Out"=w735:refnum<k24>)  [unwired: 6 in, 2 out]
                                n157 = call "XY Go.vi"("Speed"=w739, "XY In"=w729, "Gantry In"=w735) -> ("Gantry Out"=w734:refnum<k24>)  [unwired: 6 in, 2 out]
                                n158 = Delete From Array(array=w731, length=4, index=0) -> (array with subset deleted=w730:T3)  [unwired: 1 out]
                                }
                                frame True {
                                n159 = case shown="True" w758 {
                                tunnel: w768 -> [w784 w809]
                                tunnel: [w783 w808] -> w767
                                tunnel: w766 -> [w780 w807]
                                tunnel: w765 -> [w779 w806]
                                tunnel: w764 -> [w778 w804]
                                tunnel: w763 -> [w777 w803]
                                tunnel: w762 -> [w776 w802]
                                tunnel: w761 -> [w775 w801]
                                tunnel: [w770 w800] -> w760
                                tunnel: w759 -> [w769 w805]
                                tunnel: w743 -> [_ w799]
                                tunnel: w757 -> [_ w798]
                                tunnel: w756 -> [_ w797]
                                tunnel: w755 -> [_ w796]
                                tunnel: w754 -> [_ w795]
                                tunnel: w753 -> [_ w794]
                                tunnel: w752 -> [_ w793]
                                tunnel: w751 -> [_ w792]
                                tunnel: w750 -> [_ w791]
                                tunnel: w749 -> [_ w790]
                                tunnel: w748 -> [_ w789]
                                tunnel: w747 -> [_ w788]
                                tunnel: w746 -> [_ w787]
                                tunnel: w745 -> [_ w786]
                                tunnel: w744 -> [_ w785]
                                frame False {
                                n160 = call "XY Go.vi"("Speed"=w776, "XY In"=w780, "Gantry In"=w775) -> ("Gantry Out"=w774:refnum<k24>)  [unwired: 6 in, 2 out]
                                n161 = call "XY Go.vi"("Speed"=w776, "XY In"=w779, "Gantry In"=w774) -> ("Gantry Out"=w773:refnum<k24>)  [unwired: 6 in, 2 out]
                                n162 = call "XY Go.vi"("Speed"=w776, "XY In"=w778, "Gantry In"=w773) -> ("Gantry Out"=w772:refnum<k24>)  [unwired: 6 in, 2 out]
                                n163 = call "XY Go.vi"("Speed"=w776, "XY In"=w777, "Gantry In"=w772) -> ("Gantry Out"=w771:refnum<k24>)  [unwired: 6 in, 2 out]
                                n164 = call "XY Go.vi"("Speed"=w776, "XY In"=w769, "Gantry In"=w771) -> ("Gantry Out"=w770:refnum<k24>)  [unwired: 6 in, 2 out]
                                n165 = Delete From Array(array=w784, length=5, index=0) -> (array with subset deleted=w783:T3)  [unwired: 1 out]
                                }
                                frame True {
                                n166 = case shown="True" w798 {
                                tunnel: w809 -> [w825 w851]
                                tunnel: [w824 w850] -> w808
                                tunnel: w807 -> [w823 w849]
                                tunnel: w806 -> [w822 w848]
                                tunnel: w805 -> [w812 w847]
                                tunnel: w804 -> [w810 w846]
                                tunnel: w803 -> [w811 w844]
                                tunnel: w802 -> [w821 w843]
                                tunnel: w801 -> [w820 w842]
                                tunnel: [w814 w841] -> w800
                                tunnel: w799 -> [w813 w845]
                                tunnel: w797 -> [_ w840]
                                tunnel: w796 -> [_ w839]
                                tunnel: w795 -> [_ w838]
                                tunnel: w794 -> [_ w837]
                                tunnel: w793 -> [_ w836]
                                tunnel: w792 -> [_ w835]
                                tunnel: w791 -> [_ w834]
                                tunnel: w790 -> [_ w833]
                                tunnel: w789 -> [_ w832]
                                tunnel: w788 -> [_ w831]
                                tunnel: w787 -> [_ w830]
                                tunnel: w786 -> [_ w829]
                                tunnel: w785 -> [_ w828]
                                frame False {
                                n167 = call "XY Go.vi"("Speed"=w821, "XY In"=w823, "Gantry In"=w820) -> ("Gantry Out"=w819:refnum<k24>)  [unwired: 6 in, 2 out]
                                n168 = call "XY Go.vi"("Speed"=w821, "XY In"=w822, "Gantry In"=w819) -> ("Gantry Out"=w818:refnum<k24>)  [unwired: 6 in, 2 out]
                                n169 = call "XY Go.vi"("Speed"=w821, "XY In"=w810, "Gantry In"=w818) -> ("Gantry Out"=w817:refnum<k24>)  [unwired: 6 in, 2 out]
                                n170 = call "XY Go.vi"("Speed"=w821, "XY In"=w811, "Gantry In"=w817) -> ("Gantry Out"=w816:refnum<k24>)  [unwired: 6 in, 2 out]
                                n171 = call "XY Go.vi"("Speed"=w821, "XY In"=w812, "Gantry In"=w816) -> ("Gantry Out"=w815:refnum<k24>)  [unwired: 6 in, 2 out]
                                n172 = call "XY Go.vi"("Speed"=w821, "XY In"=w813, "Gantry In"=w815) -> ("Gantry Out"=w814:refnum<k24>)  [unwired: 6 in, 2 out]
                                n173 = Delete From Array(array=w825, length=6, index=0) -> (array with subset deleted=w824:T3)  [unwired: 1 out]
                                }
                                frame True {
                                n174 = case shown="True" w840 {
                                tunnel: w851 -> [w869 w884]
                                tunnel: [w868 w883] -> w850
                                tunnel: w849 -> [w867 w894]
                                tunnel: w848 -> [w866 w893]
                                tunnel: w847 -> [w852 w892]
                                tunnel: w846 -> [w854 w891]
                                tunnel: w845 -> [w853 w890]
                                tunnel: w844 -> [w855 w889]
                                tunnel: w843 -> [w865 w887]
                                tunnel: w842 -> [w864 w886]
                                tunnel: [w857 w885] -> w841
                                tunnel: w839 -> [w856 w888]
                                tunnel: w838 -> [_ w882]
                                tunnel: w837 -> [_ w881]
                                tunnel: w836 -> [_ w880]
                                tunnel: w835 -> [_ w879]
                                tunnel: w834 -> [_ w878]
                                tunnel: w833 -> [_ w877]
                                tunnel: w832 -> [_ w876]
                                tunnel: w831 -> [_ w875]
                                tunnel: w830 -> [_ w874]
                                tunnel: w829 -> [_ w873]
                                tunnel: w828 -> [_ w872]
                                frame False {
                                n175 = call "XY Go.vi"("Speed"=w865, "XY In"=w867, "Gantry In"=w864) -> ("Gantry Out"=w863:refnum<k24>)  [unwired: 6 in, 2 out]
                                n176 = call "XY Go.vi"("Speed"=w865, "XY In"=w866, "Gantry In"=w863) -> ("Gantry Out"=w862:refnum<k24>)  [unwired: 6 in, 2 out]
                                n177 = call "XY Go.vi"("Speed"=w865, "XY In"=w854, "Gantry In"=w862) -> ("Gantry Out"=w861:refnum<k24>)  [unwired: 6 in, 2 out]
                                n178 = call "XY Go.vi"("Speed"=w865, "XY In"=w855, "Gantry In"=w861) -> ("Gantry Out"=w860:refnum<k24>)  [unwired: 6 in, 2 out]
                                n179 = call "XY Go.vi"("Speed"=w865, "XY In"=w852, "Gantry In"=w860) -> ("Gantry Out"=w859:refnum<k24>)  [unwired: 6 in, 2 out]
                                n180 = call "XY Go.vi"("Speed"=w865, "XY In"=w853, "Gantry In"=w859) -> ("Gantry Out"=w858:refnum<k24>)  [unwired: 6 in, 2 out]
                                n181 = call "XY Go.vi"("Speed"=w865, "XY In"=w856, "Gantry In"=w858) -> ("Gantry Out"=w857:refnum<k24>)  [unwired: 6 in, 2 out]
                                n182 = Delete From Array(array=w869, length=7, index=0) -> (array with subset deleted=w868:T3)  [unwired: 1 out]
                                }
                                frame True {
                                n183 = case shown="True" w881 {
                                tunnel: w894 -> [w916 w936]
                                tunnel: w893 -> [w915 w935]
                                tunnel: w892 -> [w896 w934]
                                tunnel: w891 -> [w898 w933]
                                tunnel: w890 -> [w895 w932]
                                tunnel: w889 -> [w897 w931]
                                tunnel: w888 -> [w914 w930]
                                tunnel: w887 -> [w913 w928]
                                tunnel: w886 -> [w912 w927]
                                tunnel: [w904 w926] -> w885
                                tunnel: w884 -> [w901 w938]
                                tunnel: [w900 w937] -> w883
                                tunnel: w882 -> [w899 w929]
                                tunnel: w880 -> [_ w925]
                                tunnel: w879 -> [_ w924]
                                tunnel: w878 -> [_ w923]
                                tunnel: w877 -> [_ w922]
                                tunnel: w876 -> [_ w921]
                                tunnel: w875 -> [_ w920]
                                tunnel: w874 -> [_ w919]
                                tunnel: w873 -> [_ w918]
                                tunnel: w872 -> [_ w917]
                                frame False {
                                n184 = call "XY Go.vi"("Speed"=w913, "XY In"=w916, "Gantry In"=w912) -> ("Gantry Out"=w911:refnum<k24>)  [unwired: 6 in, 2 out]
                                n185 = call "XY Go.vi"("Speed"=w913, "XY In"=w915, "Gantry In"=w911) -> ("Gantry Out"=w910:refnum<k24>)  [unwired: 6 in, 2 out]
                                n186 = call "XY Go.vi"("Speed"=w913, "XY In"=w898, "Gantry In"=w910) -> ("Gantry Out"=w909:refnum<k24>)  [unwired: 6 in, 2 out]
                                n187 = call "XY Go.vi"("Speed"=w913, "XY In"=w897, "Gantry In"=w909) -> ("Gantry Out"=w908:refnum<k24>)  [unwired: 6 in, 2 out]
                                n188 = call "XY Go.vi"("Speed"=w913, "XY In"=w896, "Gantry In"=w908) -> ("Gantry Out"=w907:refnum<k24>)  [unwired: 6 in, 2 out]
                                n189 = call "XY Go.vi"("Speed"=w913, "XY In"=w895, "Gantry In"=w907) -> ("Gantry Out"=w906:refnum<k24>)  [unwired: 6 in, 2 out]
                                n190 = call "XY Go.vi"("Speed"=w913, "XY In"=w914, "Gantry In"=w906) -> ("Gantry Out"=w905:refnum<k24>)  [unwired: 6 in, 2 out]
                                n191 = call "XY Go.vi"("Speed"=w913, "XY In"=w899, "Gantry In"=w905) -> ("Gantry Out"=w904:refnum<k24>)  [unwired: 6 in, 2 out]
                                n192 = Delete From Array(array=w901, length=8, index=0) -> (array with subset deleted=w900:T3)  [unwired: 1 out]
                                }
                                frame True {
                                n193 = case shown="True" w924 {
                                tunnel: w938 -> [w962 w983]
                                tunnel: [w961 w982] -> w937
                                tunnel: w936 -> [w958 w981]
                                tunnel: w935 -> [w957 w980]
                                tunnel: w934 -> [w942 w979]
                                tunnel: w933 -> [w941 w978]
                                tunnel: w932 -> [w940 w977]
                                tunnel: w931 -> [w939 w976]
                                tunnel: w930 -> [w956 w975]
                                tunnel: w929 -> [w955 w974]
                                tunnel: w928 -> [w954 w972]
                                tunnel: w927 -> [w953 w971]
                                tunnel: [w944 w970] -> w926
                                tunnel: w925 -> [w943 w973]
                                tunnel: w923 -> [_ w969]
                                tunnel: w922 -> [_ w968]
                                tunnel: w921 -> [_ w967]
                                tunnel: w920 -> [_ w966]
                                tunnel: w919 -> [_ w965]
                                tunnel: w918 -> [_ w964]
                                tunnel: w917 -> [_ w963]
                                frame False {
                                n194 = call "XY Go.vi"("Speed"=w954, "XY In"=w958, "Gantry In"=w953) -> ("Gantry Out"=w952:refnum<k24>)  [unwired: 6 in, 2 out]
                                n195 = call "XY Go.vi"("Speed"=w954, "XY In"=w957, "Gantry In"=w952) -> ("Gantry Out"=w951:refnum<k24>)  [unwired: 6 in, 2 out]
                                n196 = call "XY Go.vi"("Speed"=w954, "XY In"=w941, "Gantry In"=w951) -> ("Gantry Out"=w950:refnum<k24>)  [unwired: 6 in, 2 out]
                                n197 = call "XY Go.vi"("Speed"=w954, "XY In"=w939, "Gantry In"=w950) -> ("Gantry Out"=w949:refnum<k24>)  [unwired: 6 in, 2 out]
                                n198 = call "XY Go.vi"("Speed"=w954, "XY In"=w942, "Gantry In"=w949) -> ("Gantry Out"=w948:refnum<k24>)  [unwired: 6 in, 2 out]
                                n199 = call "XY Go.vi"("Speed"=w954, "XY In"=w940, "Gantry In"=w948) -> ("Gantry Out"=w947:refnum<k24>)  [unwired: 6 in, 2 out]
                                n200 = call "XY Go.vi"("Speed"=w954, "XY In"=w956, "Gantry In"=w947) -> ("Gantry Out"=w946:refnum<k24>)  [unwired: 6 in, 2 out]
                                n201 = call "XY Go.vi"("Speed"=w954, "XY In"=w955, "Gantry In"=w946) -> ("Gantry Out"=w945:refnum<k24>)  [unwired: 6 in, 2 out]
                                n202 = call "XY Go.vi"("Speed"=w954, "XY In"=w943, "Gantry In"=w945) -> ("Gantry Out"=w944:refnum<k24>)  [unwired: 6 in, 2 out]
                                n203 = Delete From Array(array=w962, length=9, index=0) -> (array with subset deleted=w961:T3)  [unwired: 1 out]
                                }
                                frame True {
                                n204 = case shown="True" w968 {
                                tunnel: w983 -> [w1009 w1029]
                                tunnel: [w1006 w1028] -> w982
                                tunnel: w981 -> [w1005 w1025]
                                tunnel: w980 -> [w1004 w1024]
                                tunnel: w979 -> [w987 w1023]
                                tunnel: w978 -> [w986 w1022]
                                tunnel: w977 -> [w985 w1021]
                                tunnel: w976 -> [w984 w1020]
                                tunnel: w975 -> [w1003 w1019]
                                tunnel: w974 -> [w1002 w1018]
                                tunnel: w973 -> [w1001 w1017]
                                tunnel: w972 -> [w1000 w1015]
                                tunnel: w971 -> [w999 w1027]
                                tunnel: [w989 w1026] -> w970
                                tunnel: w969 -> [w988 w1016]
                                tunnel: w967 -> [_ w1014]
                                tunnel: w966 -> [_ w1013]
                                tunnel: w965 -> [_ w1012]
                                tunnel: w964 -> [_ w1011]
                                tunnel: w963 -> [_ w1010]
                                frame False {
                                n205 = call "XY Go.vi"("Speed"=w1000, "XY In"=w1005, "Gantry In"=w999) -> ("Gantry Out"=w998:refnum<k24>)  [unwired: 6 in, 2 out]
                                n206 = Delete From Array(array=w1009, length=10, index=0) -> (array with subset deleted=w1006:T3)  [unwired: 1 out]
                                n207 = call "XY Go.vi"("Speed"=w1000, "XY In"=w1004, "Gantry In"=w998) -> ("Gantry Out"=w997:refnum<k24>)  [unwired: 6 in, 2 out]
                                n208 = call "XY Go.vi"("Speed"=w1000, "XY In"=w986, "Gantry In"=w997) -> ("Gantry Out"=w996:refnum<k24>)  [unwired: 6 in, 2 out]
                                n209 = call "XY Go.vi"("Speed"=w1000, "XY In"=w984, "Gantry In"=w996) -> ("Gantry Out"=w995:refnum<k24>)  [unwired: 6 in, 2 out]
                                n210 = call "XY Go.vi"("Speed"=w1000, "XY In"=w987, "Gantry In"=w995) -> ("Gantry Out"=w994:refnum<k24>)  [unwired: 6 in, 2 out]
                                n211 = call "XY Go.vi"("Speed"=w1000, "XY In"=w985, "Gantry In"=w994) -> ("Gantry Out"=w993:refnum<k24>)  [unwired: 6 in, 2 out]
                                n212 = call "XY Go.vi"("Speed"=w1000, "XY In"=w1003, "Gantry In"=w993) -> ("Gantry Out"=w992:refnum<k24>)  [unwired: 6 in, 2 out]
                                n213 = call "XY Go.vi"("Speed"=w1000, "XY In"=w1002, "Gantry In"=w992) -> ("Gantry Out"=w991:refnum<k24>)  [unwired: 6 in, 2 out]
                                n214 = call "XY Go.vi"("Speed"=w1000, "XY In"=w1001, "Gantry In"=w991) -> ("Gantry Out"=w990:refnum<k24>)  [unwired: 6 in, 2 out]
                                n215 = call "XY Go.vi"("Speed"=w1000, "XY In"=w988, "Gantry In"=w990) -> ("Gantry Out"=w989:refnum<k24>)  [unwired: 6 in, 2 out]
                                }
                                frame True {
                                n216 = case shown="True" w1013 {
                                tunnel: w1029 -> [w1057 w1076]
                                tunnel: [w1054 w1075] -> w1028
                                tunnel: w1027 -> [w1053 w1063]
                                tunnel: [w1042 w1062] -> w1026
                                tunnel: w1025 -> [w1041 w1074]
                                tunnel: w1024 -> [w1040 w1073]
                                tunnel: w1023 -> [w1034 w1072]
                                tunnel: w1022 -> [w1032 w1071]
                                tunnel: w1021 -> [w1033 w1070]
                                tunnel: w1020 -> [w1035 w1069]
                                tunnel: w1019 -> [w1039 w1068]
                                tunnel: w1018 -> [w1038 w1067]
                                tunnel: w1017 -> [w1030 w1066]
                                tunnel: w1016 -> [w1031 w1065]
                                tunnel: w1015 -> [w1037 w1058]
                                tunnel: w1014 -> [w1036 w1064]
                                tunnel: w1012 -> [_ w1061]
                                tunnel: w1011 -> [_ w1060]
                                tunnel: w1010 -> [_ w1059]
                                frame False {
                                n217 = call "XY Go.vi"("Speed"=w1037, "XY In"=w1041, "Gantry In"=w1053) -> ("Gantry Out"=w1052:refnum<k24>)  [unwired: 6 in, 2 out]
                                n218 = Delete From Array(array=w1057, length=11, index=0) -> (array with subset deleted=w1054:T3)  [unwired: 1 out]
                                n219 = call "XY Go.vi"("Speed"=w1037, "XY In"=w1040, "Gantry In"=w1052) -> ("Gantry Out"=w1051:refnum<k24>)  [unwired: 6 in, 2 out]
                                n220 = call "XY Go.vi"("Speed"=w1037, "XY In"=w1032, "Gantry In"=w1051) -> ("Gantry Out"=w1050:refnum<k24>)  [unwired: 6 in, 2 out]
                                n221 = call "XY Go.vi"("Speed"=w1037, "XY In"=w1035, "Gantry In"=w1050) -> ("Gantry Out"=w1049:refnum<k24>)  [unwired: 6 in, 2 out]
                                n222 = call "XY Go.vi"("Speed"=w1037, "XY In"=w1034, "Gantry In"=w1049) -> ("Gantry Out"=w1048:refnum<k24>)  [unwired: 6 in, 2 out]
                                n223 = call "XY Go.vi"("Speed"=w1037, "XY In"=w1033, "Gantry In"=w1048) -> ("Gantry Out"=w1047:refnum<k24>)  [unwired: 6 in, 2 out]
                                n224 = call "XY Go.vi"("Speed"=w1037, "XY In"=w1039, "Gantry In"=w1047) -> ("Gantry Out"=w1046:refnum<k24>)  [unwired: 6 in, 2 out]
                                n225 = call "XY Go.vi"("Speed"=w1037, "XY In"=w1038, "Gantry In"=w1046) -> ("Gantry Out"=w1045:refnum<k24>)  [unwired: 6 in, 2 out]
                                n226 = call "XY Go.vi"("Speed"=w1037, "XY In"=w1030, "Gantry In"=w1045) -> ("Gantry Out"=w1044:refnum<k24>)  [unwired: 6 in, 2 out]
                                n227 = call "XY Go.vi"("Speed"=w1037, "XY In"=w1031, "Gantry In"=w1044) -> ("Gantry Out"=w1043:refnum<k24>)  [unwired: 6 in, 2 out]
                                n228 = call "XY Go.vi"("Speed"=w1037, "XY In"=w1036, "Gantry In"=w1043) -> ("Gantry Out"=w1042:refnum<k24>)  [unwired: 6 in, 2 out]
                                }
                                frame True {
                                n229 = case shown="False" w1060 {
                                tunnel: w1076 -> [w1105 w1138]
                                tunnel: [w1104 w1137] -> w1075
                                tunnel: w1074 -> [w1103 w1136]
                                tunnel: w1073 -> [w1102 w1135]
                                tunnel: w1072 -> [w1079 w1110]
                                tunnel: w1071 -> [w1077 w1108]
                                tunnel: w1070 -> [w1078 w1111]
                                tunnel: w1069 -> [w1080 w1109]
                                tunnel: w1068 -> [w1101 w1134]
                                tunnel: w1067 -> [w1100 w1133]
                                tunnel: w1066 -> [w1099 w1132]
                                tunnel: w1065 -> [w1098 w1131]
                                tunnel: w1064 -> [w1097 w1130]
                                tunnel: w1063 -> [w1096 w1127]
                                tunnel: [w1084 w1114] -> w1062
                                tunnel: w1061 -> [w1083 w1129]
                                tunnel: w1059 -> [_ w1128]
                                tunnel: w1058 -> [w1081 w1113]
                                frame False {
                                w1082 = FALSE
                                n230 = call "XY Go.vi"("return immediately"=w1082, "Speed"=w1081, "XY In"=w1103, "Gantry In"=w1096) -> ("Gantry Out"=w1095:refnum<k24>)  [unwired: 5 in, 2 out]
                                n231 = Delete From Array(array=w1105, length=12, index=0) -> (array with subset deleted=w1104:T3)  [unwired: 1 out]
                                n232 = call "XY Go.vi"("return immediately"=w1082, "Speed"=w1081, "XY In"=w1102, "Gantry In"=w1095) -> ("Gantry Out"=w1094:refnum<k24>)  [unwired: 5 in, 2 out]
                                n233 = call "XY Go.vi"("return immediately"=w1082, "Speed"=w1081, "XY In"=w1077, "Gantry In"=w1094) -> ("Gantry Out"=w1093:refnum<k24>)  [unwired: 5 in, 2 out]
                                n234 = call "XY Go.vi"("return immediately"=w1082, "Speed"=w1081, "XY In"=w1080, "Gantry In"=w1093) -> ("Gantry Out"=w1092:refnum<k24>)  [unwired: 5 in, 2 out]
                                n235 = call "XY Go.vi"("return immediately"=w1082, "Speed"=w1081, "XY In"=w1079, "Gantry In"=w1092) -> ("Gantry Out"=w1091:refnum<k24>)  [unwired: 5 in, 2 out]
                                n236 = call "XY Go.vi"("return immediately"=w1082, "Speed"=w1081, "XY In"=w1078, "Gantry In"=w1091) -> ("Gantry Out"=w1090:refnum<k24>)  [unwired: 5 in, 2 out]
                                n237 = call "XY Go.vi"("return immediately"=w1082, "Speed"=w1081, "XY In"=w1101, "Gantry In"=w1090) -> ("Gantry Out"=w1089:refnum<k24>)  [unwired: 5 in, 2 out]
                                n238 = call "XY Go.vi"("return immediately"=w1082, "Speed"=w1081, "XY In"=w1100, "Gantry In"=w1089) -> ("Gantry Out"=w1088:refnum<k24>)  [unwired: 5 in, 2 out]
                                n239 = call "XY Go.vi"("return immediately"=w1082, "Speed"=w1081, "XY In"=w1099, "Gantry In"=w1088) -> ("Gantry Out"=w1087:refnum<k24>)  [unwired: 5 in, 2 out]
                                n240 = call "XY Go.vi"("return immediately"=w1082, "Speed"=w1081, "XY In"=w1098, "Gantry In"=w1087) -> ("Gantry Out"=w1086:refnum<k24>)  [unwired: 5 in, 2 out]
                                n241 = call "XY Go.vi"("return immediately"=w1082, "Speed"=w1081, "XY In"=w1097, "Gantry In"=w1086) -> ("Gantry Out"=w1085:refnum<k24>)  [unwired: 5 in, 2 out]
                                n242 = call "XY Go.vi"("return immediately"=w1082, "Speed"=w1081, "XY In"=w1083, "Gantry In"=w1085) -> ("Gantry Out"=w1084:refnum<k24>)  [unwired: 5 in, 2 out]
                                }
                                frame True {
                                w1112 = FALSE
                                n243 = Delete From Array(array=w1138, length=13, index=0) -> (array with subset deleted=w1137:T3)  [unwired: 1 out]
                                n244 = call "XY Go.vi"("return immediately"=w1112, "Speed"=w1113, "XY In"=w1136, "Gantry In"=w1127) -> ("Gantry Out"=w1126:refnum<k24>)  [unwired: 5 in, 2 out]
                                n245 = call "XY Go.vi"("return immediately"=w1112, "Speed"=w1113, "XY In"=w1135, "Gantry In"=w1126) -> ("Gantry Out"=w1125:refnum<k24>)  [unwired: 5 in, 2 out]
                                n246 = call "XY Go.vi"("return immediately"=w1112, "Speed"=w1113, "XY In"=w1108, "Gantry In"=w1125) -> ("Gantry Out"=w1124:refnum<k24>)  [unwired: 5 in, 2 out]
                                n247 = call "XY Go.vi"("return immediately"=w1112, "Speed"=w1113, "XY In"=w1109, "Gantry In"=w1124) -> ("Gantry Out"=w1123:refnum<k24>)  [unwired: 5 in, 2 out]
                                n248 = call "XY Go.vi"("return immediately"=w1112, "Speed"=w1113, "XY In"=w1110, "Gantry In"=w1123) -> ("Gantry Out"=w1122:refnum<k24>)  [unwired: 5 in, 2 out]
                                n249 = call "XY Go.vi"("return immediately"=w1112, "Speed"=w1113, "XY In"=w1111, "Gantry In"=w1122) -> ("Gantry Out"=w1121:refnum<k24>)  [unwired: 5 in, 2 out]
                                n250 = call "XY Go.vi"("return immediately"=w1112, "Speed"=w1113, "XY In"=w1134, "Gantry In"=w1121) -> ("Gantry Out"=w1120:refnum<k24>)  [unwired: 5 in, 2 out]
                                n251 = call "XY Go.vi"("return immediately"=w1112, "Speed"=w1113, "XY In"=w1133, "Gantry In"=w1120) -> ("Gantry Out"=w1119:refnum<k24>)  [unwired: 5 in, 2 out]
                                n252 = call "XY Go.vi"("return immediately"=w1112, "Speed"=w1113, "XY In"=w1132, "Gantry In"=w1119) -> ("Gantry Out"=w1118:refnum<k24>)  [unwired: 5 in, 2 out]
                                n253 = call "XY Go.vi"("return immediately"=w1112, "Speed"=w1113, "XY In"=w1131, "Gantry In"=w1118) -> ("Gantry Out"=w1117:refnum<k24>)  [unwired: 5 in, 2 out]
                                n254 = call "XY Go.vi"("return immediately"=w1112, "Speed"=w1113, "XY In"=w1130, "Gantry In"=w1117) -> ("Gantry Out"=w1116:refnum<k24>)  [unwired: 5 in, 2 out]
                                n255 = call "XY Go.vi"("return immediately"=w1112, "Speed"=w1113, "XY In"=w1129, "Gantry In"=w1116) -> ("Gantry Out"=w1115:refnum<k24>)  [unwired: 5 in, 2 out]
                                n256 = call "XY Go.vi"("return immediately"=w1112, "Speed"=w1113, "XY In"=w1128, "Gantry In"=w1115) -> ("Gantry Out"=w1114:refnum<k24>)  [unwired: 5 in, 2 out]
                                }
                                }
                                }
                                }
                                }
                                }
                                }
                                }
                                }
                                }
                                }
                                }
                                }
                                }
                                }
                                }
                                }
                              }
                            }
                          }
                        }
                      }
                    }
                  }
                  n257 = flat-sequence {
                    tunnel: [w1141] -> w610
                    tunnel: [w1145] -> w607
                    tunnel: [w1144] -> w604
                    tunnel: w609 -> [w1146]
                    tunnel: w606 -> [w1145]
                    tunnel: w603 -> [w1144]
                    tunnel: w598 -> [w1142]
                    tunnel: w571 -> [w1141]
                    tunnel: [w1150] -> w611
                    tunnel: w610 -> [w1149]
                    tunnel: [w1148] -> w608
                    tunnel: w607 -> [w1148]
                    tunnel: [w1147] -> w605
                    tunnel: w604 -> [w1147]
                    frame #0 {
                      n258 = Subtract(x=w1146, y=w1142) -> (x-y=w1143:i32)
                      n259 = Wait (ms)(milliseconds to wait=w1143) -> ()  [unwired: 1 out]
                    }
                    frame #1 {
                      n260 = call "Dispense.vi"("Dispenser In"=w1149) -> ("Dispenser Out"=w1150:refnum<visa-resource-name>)  [unwired: 9 in, 1 out]
                    }
                  }
                }
                frame #3 {
                  n261 = Negate(x=w1155) -> (-x=w1154:dbl)
                  n262 = call "Z Go.vi"("Increment"=TRUE, "Return Immediately"=FALSE, "Speed In"=w1153, "Position In"=w1154, "Gantry In"=w1156) -> ("Gantry Out"=w1158:refnum<k24>)  [unwired: 3 in, 3 out]
                }
              }
            }
            frame "Arc" {
              n263 = Index Array(array=w1188) -> (element #1=w1167:dbl[], element #2=w1182:dbl[])  [unwired: 4 in]
              n264 = flat-sequence {
                tunnel: [w1206] -> w1198
                tunnel: w1190 -> [w1205]
                tunnel: w1189 -> [w1204]
                tunnel: w1167 -> [w1203]
                tunnel: w1187 -> [w1202]
                tunnel: [w1201] -> w1174
                tunnel: w1173 -> [w1200]
                tunnel: w1172 -> [w1199]
                tunnel: w1198 -> [w1231]
                tunnel: [w1232] -> w1197
                tunnel: [w1228] -> w1196
                tunnel: [w1225] -> w1195
                tunnel: [w1222] -> w1194
                tunnel: w1186 -> [w1221]
                tunnel: w1185 -> [w1220]
                tunnel: w1184 -> [w1219]
                tunnel: w1183 -> [w1218]
                tunnel: w1174 -> [w1217]
                tunnel: w1197 -> [w1275]
                tunnel: [w1276] -> w1193
                tunnel: w1196 -> [w1266]
                tunnel: w1195 -> [w1279]
                tunnel: [w1279] -> w1192
                tunnel: w1194 -> [w1278]
                tunnel: [w1278] -> w1191
                tunnel: w1182 -> [w1269]
                tunnel: w1181 -> [w1268]
                tunnel: w1180 -> [w1270]
                tunnel: w1179 -> [w1272]
                tunnel: w1178 -> [w1277]
                tunnel: [w1267] -> w1175
                tunnel: w1171 -> [w1273]
                tunnel: w1170 -> [w1265]
                tunnel: w1169 -> [w1264]
                tunnel: w1168 -> [w1263]
                tunnel: w1167 -> [w1262]
                tunnel: w1166 -> [w1261]
                tunnel: w1165 -> [w1260]
                tunnel: w1164 -> [w1259]
                tunnel: w1163 -> [w1258]
                tunnel: w1162 -> [w1257]
                tunnel: w1161 -> [w1256]
                tunnel: [w1255] -> w1160
                tunnel: w1159 -> [w1254]
                tunnel: [w1388] -> w1177
                tunnel: w1193 -> [w1387]
                tunnel: [w1387] -> w1176
                tunnel: w1192 -> [w1385]
                tunnel: w1191 -> [w1383]
                tunnel: w1175 -> [w1386]
                frame #0 {
                  n265 = call "Pressure.vi"("Pressure"=w1199, "VISA resource name"=w1200) -> ("VISA resource name out"=w1201:refnum<visa-resource-name>)  [unwired: 8 in, 1 out]
                  n266 = case shown="True" w1205 {
                    tunnel: [w1211 w1214] -> w1206
                    tunnel: w1204 -> [w1210 w1213]
                    tunnel: w1203 -> [w1209 w1212]
                    tunnel: w1202 -> [w1208 _]
                    frame False {
                      n267 = call "XY Go.vi"("return immediately"=FALSE, "Speed"=w1208, "XY In"=w1209, "Gantry In"=w1210) -> ("Gantry Out"=w1211:refnum<k24>)  [unwired: 5 in, 2 out]
                    }
                    frame True {
                      n268 = call "ClearXYZTheta Go.vi"("XYZTheta In"=w1212, "Gantry In"=w1213) -> ("Gantry Out"=w1214:refnum<k24>)  [unwired: 7 in, 2 out]
                    }
                  }
                }
                frame #1 {
                  n269 = flat-sequence {
                    tunnel: w1231 -> [w1241]
                    tunnel: [w1239] -> w1230
                    tunnel: [w1238] -> w1227
                    tunnel: [w1237] -> w1226
                    tunnel: w1219 -> [w1236]
                    tunnel: w1218 -> [w1235]
                    tunnel: w1217 -> [w1233]
                    tunnel: [w1233] -> w1216
                    tunnel: w1230 -> [w1248]
                    tunnel: [w1248] -> w1229
                    tunnel: w1227 -> [w1247]
                    tunnel: w1226 -> [w1246]
                    tunnel: [w1247] -> w1224
                    tunnel: [w1246] -> w1223
                    tunnel: w1221 -> [w1245]
                    tunnel: w1220 -> [w1244]
                    tunnel: w1216 -> [w1243]
                    tunnel: [w1243] -> w1215
                    tunnel: [w1253] -> w1232
                    tunnel: w1229 -> [w1252]
                    tunnel: [w1252] -> w1228
                    tunnel: [w1251] -> w1225
                    tunnel: w1224 -> [w1251]
                    tunnel: w1223 -> [w1250]
                    tunnel: [w1250] -> _
                    tunnel: [w1250] -> w1222
                    tunnel: w1215 -> [w1249]
                    frame #0 {
                      n270 = call "Z Go.vi"("Increment"=TRUE, "Return Immediately"=TRUE, "Speed In"=w1235, "Position In"=w1236, "Gantry In"=w1241) -> ("Speed Out"=w1237:dbl, "Position Out"=w1238:dbl, "Gantry Out"=w1239:refnum<k24>)  [unwired: 3 in, 1 out]
                    }
                    frame #1 {
                      n271 = Subtract(x=w1245, y=w1244) -> (x-y=w1242:i32)
                      n272 = Wait (ms)(milliseconds to wait=w1242) -> ()  [unwired: 1 out]
                    }
                    frame #2 {
                      n273 = call "Dispense.vi"("Dispenser In"=w1249) -> ("Dispenser Out"=w1253:refnum<visa-resource-name>)  [unwired: 9 in, 1 out]
                    }
                  }
                }
                frame #2 {
                  n274 = flat-sequence {
                    tunnel: [w1376] -> w1274
                    tunnel: w1277 -> [w1378]
                    tunnel: w1275 -> [w1376]
                    tunnel: w1273 -> [w1375]
                    tunnel: [w1380] -> w1276
                    tunnel: w1274 -> [w1379]
                    frame #0 {
                      n275 = Subtract(x=w1378, y=w1375) -> (x-y=w1377:i32)
                      n276 = Wait (ms)(milliseconds to wait=w1377) -> ()  [unwired: 1 out]
                    }
                    frame #1 {
                      n277 = call "Dispense.vi"("Dispenser In"=w1379) -> ("Dispenser Out"=w1380:refnum<visa-resource-name>)  [unwired: 9 in, 1 out]
                    }
                  }
                  n278 = case shown="True" w1259 {
                    tunnel: w1272 -> [w1290 w1305]
                    tunnel: FALSE ("return immediately") -> [w1289 _]
                    tunnel: w1270 -> [w1288 w1304]
                    tunnel: w1269 -> [w1287 w1306]
                    tunnel: w1268 -> [w1286 w1307]
                    tunnel: [w1285 w1294] -> w1267
                    tunnel: w1266 -> [w1284 w1295]
                    tunnel: w1265 -> [_ w1303]
                    tunnel: w1264 -> [_ w1302]
                    tunnel: w1263 -> [_ w1301]
                    tunnel: w1262 -> [_ w1300]
                    tunnel: w1261 -> [_ w1299]
                    tunnel: w1260 -> [_ w1298]
                    tunnel: w1258 -> [_ w1297]
                    tunnel: w1257 -> [_ w1296]
                    tunnel: w1256 -> [w1283 w1293]
                    tunnel: [w1280 w1292] -> w1255
                    tunnel: w1254 -> [_ w1291]
                    frame False {
                      n279 = call "Circular.vi"("Direction"=w1290, "return immediately"=w1289, "Speed"=w1288, "XY End"=w1287, "XY Center"=w1286, "Gantry In"=w1284) -> ("Gantry Out"=w1285:refnum<k24>)  [unwired: 4 in, 1 out]
                      n280 = Delete From Array(array=w1283, length=1, index=0) -> (array with subset deleted=w1280:T3)  [unwired: 1 out]
                    }
                    frame True {
                      n281 = case shown="True" w1297 {
                        tunnel: w1307 -> [w1321 w1335]
                        tunnel: w1306 -> [w1320 w1334]
                        tunnel: w1305 -> [w1319 w1325]
                        tunnel: w1304 -> [w1318 w1326]
                        tunnel: w1303 -> [w1316 w1336]
                        tunnel: w1302 -> [w1315 w1337]
                        tunnel: w1301 -> [_ w1333]
                        tunnel: w1300 -> [_ w1332]
                        tunnel: w1299 -> [_ w1331]
                        tunnel: w1298 -> [_ w1330]
                        tunnel: w1296 -> [_ w1329]
                        tunnel: w1295 -> [w1314 w1328]
                        tunnel: [w1312 w1327] -> w1294
                        tunnel: w1293 -> [w1311 w1324]
                        tunnel: [w1310 w1323] -> w1292
                        tunnel: w1291 -> [_ w1322]
                        frame False {
                          w1317 = FALSE
                          n282 = call "Circular.vi"("Direction"=w1319, "return immediately"=w1317, "Speed"=w1318, "XY End"=w1320, "XY Center"=w1321, "Gantry In"=w1314) -> ("Gantry Out"=w1313:refnum<k24>)  [unwired: 4 in, 1 out]
                          n283 = call "Circular.vi"("Direction"=w1319, "return immediately"=w1317, "Speed"=w1318, "XY End"=w1316, "XY Center"=w1315, "Gantry In"=w1313) -> ("Gantry Out"=w1312:refnum<k24>)  [unwired: 4 in, 1 out]
                          n284 = Delete From Array(array=w1311, length=2, index=0) -> (array with subset deleted=w1310:T3)  [unwired: 1 out]
                        }
                        frame True {
                          n285 = case shown="True" w1329 {
                            tunnel: w1337 -> [w1353 w1374]
                            tunnel: w1336 -> [w1350 w1373]
                            tunnel: w1335 -> [w1352 w1372]
                            tunnel: w1334 -> [w1351 w1371]
                            tunnel: w1333 -> [w1354 w1370]
                            tunnel: w1332 -> [_ _]
                            tunnel: w1331 -> [_ w1369]
                            tunnel: w1330 -> [_ w1368]
                            tunnel: w1328 -> [w1349 w1367]
                            tunnel: [w1346 w1363] -> w1327
                            tunnel: w1326 -> [w1345 w1362]
                            tunnel: w1325 -> [w1344 w1361]
                            tunnel: w1324 -> [w1342 w1359]
                            tunnel: [w1341 w1358] -> w1323
                            tunnel: w1322 -> [w1338 w1355]
                            frame False {
                              w1343 = FALSE
                              n286 = call "Circular.vi"("Direction"=w1344, "return immediately"=w1343, "Speed"=w1345, "XY End"=w1351, "XY Center"=w1352, "Gantry In"=w1349) -> ("Gantry Out"=w1348:refnum<k24>)  [unwired: 4 in, 1 out]
                              n287 = call "Circular.vi"("Direction"=w1344, "return immediately"=w1343, "Speed"=w1345, "XY End"=w1350, "XY Center"=w1353, "Gantry In"=w1348) -> ("Gantry Out"=w1347:refnum<k24>)  [unwired: 4 in, 1 out]
                              n288 = call "Circular.vi"("Direction"=w1344, "return immediately"=w1343, "Speed"=w1345, "XY End"=w1338, "XY Center"=w1354, "Gantry In"=w1347) -> ("Gantry Out"=w1346:refnum<k24>)  [unwired: 4 in, 1 out]
                              n289 = Delete From Array(array=w1342, length=3, index=0) -> (array with subset deleted=w1341:T3)  [unwired: 1 out]
                            }
                            frame True {
                              w1360 = FALSE
                              n290 = Delete From Array(array=w1359, length=4, index=0) -> (array with subset deleted=w1358:T3)  [unwired: 1 out]
                              n291 = call "Circular.vi"("Direction"=w1361, "return immediately"=w1360, "Speed"=w1362, "XY End"=w1371, "XY Center"=w1372, "Gantry In"=w1367) -> ("Gantry Out"=w1366:refnum<k24>)  [unwired: 4 in, 1 out]
                              n292 = call "Circular.vi"("Direction"=w1361, "return immediately"=w1360, "Speed"=w1362, "XY End"=w1373, "XY Center"=w1374, "Gantry In"=w1366) -> ("Gantry Out"=w1365:refnum<k24>)  [unwired: 4 in, 1 out]
                              n293 = call "Circular.vi"("Direction"=w1361, "return immediately"=w1360, "Speed"=w1362, "XY End"=w1355, "XY Center"=w1370, "Gantry In"=w1365) -> ("Gantry Out"=w1364:refnum<k24>)  [unwired: 4 in, 1 out]
                              n294 = call "Circular.vi"("Direction"=w1361, "return immediately"=w1360, "Speed"=w1362, "XY End"=w1368, "XY Center"=w1369, "Gantry In"=w1364) -> ("Gantry Out"=w1363:refnum<k24>)  [unwired: 4 in, 1 out]
                            }
                          }
                        }
                      }
                    }
                  }
                }
                frame #3 {
                  n295 = Negate(x=w1385) -> (-x=w1384:dbl)
                  n296 = call "Z Go.vi"("Increment"=TRUE, "Return Immediately"=FALSE, "Speed In"=w1383, "Position In"=w1384, "Gantry In"=w1386) -> ("Gantry Out"=w1388:refnum<k24>)  [unwired: 3 in, 3 out]
                }
              }
            }
          }
          n297 = Array Size(array=w111) -> (size(s)=w112:i32)
          n298 = Equal To 0?(x=w112) -> (x = 0?=w113:bool)
        }
        n299 = in-place-cluster #1("Gantry"=w22, "Dispenser"=w18) -> (w9:T2)
      }
    }
    frame Error {
    }
  }
  "error out" <- w2
  "Sensor Dispense out" <- w5
  "Control Out" <- w3
